vi "ME_acquire_17_DeltaForce_Daq_SteppingMode.vi"() -> ()   [LabVIEW 2015]
doc: "Use this template to build a producer/consumer design pattern. Use this template when you need to execute a process, such as data analysis, when a data source, such as a triggered acquisition, produces data at an uneven rate and you need to execute the process when the data becomes available."
uses:
  Mode.ctl
  oxford_driver/Oxford Drivers/BUSGEN.LLB/OxfordAddress.ctl
  <vilib>/Analysis/baseanly.llb/Mean (DBL).vi
  <vilib>/DAQmx/read.llb/DAQmx Read (Analog 1D DBL 1Chan NSamp).vi
  <vilib>/DAQmx/create/channels.llb/DAQmx Create Channel (AI-Voltage-Basic).vi
  <vilib>/DAQmx/configure/timing.llb/DAQmx Timing (Sample Clock).vi
  <vilib>/Utility/file.llb/Write Delimited Spreadsheet (DBL).vi
  <vilib>/DAQmx/miscellaneous.llb/DAQmx Fill In Error Info.vi
  <vilib>/express/express arith-compare/Formula/XNode/ExpressFormulaBlockNode.xnode
  <vilib>/Analysis/NI_AALBase.lvlib
panel:
  in  "First Offset?":bool
  out "Last2":dbl
  out "Actual2":dbl
  out "Up/Down":bool
  out "T array":dbl[](array[numeric])
  out "Averaged I(T)":dbl[][](array[numeric])
  in  "Averaged P(T)":dbl[][](array[numeric])
  out "remaining elements 2":T1(array[cluster])
  out "Actual mean":dbl format="%0.6f"
  in  "Averaged dt":dbl[][](array[numeric])
  in  "Averaged P(B)":dbl[][](array[numeric])
  out "LockInR":dbl
  out "deltaUaux":dbl
  out "Actual Voltage (V)":dbl caption="Actual AuxV" step=0.1
  in  "Stop":bool
  out "SaveSweep":bool=TRUE
  out "Measurement File_dn":path
  out "Measurement File_up":path
  out "Measurement File_average":path
  out "Actual Polarization":dbl
  in  "Reset IB?":bool
  in  "First?":bool
  in  "Save Period":dbl=1.0
  out "Averaged I(B)":dbl[][](array[numeric])
  out "P(uC/mm^2)":dbl[](array[numeric])
  in  "Sweep":bool
  out "Offset array":dbl[](array[numeric])
  in  "stop 2":bool
  in  "dB":dbl=0.005
  out "appended array":dbl[][](array[numeric])
  out "Actual B Field (T)":dbl
  out "Actual Temperature (K)":dbl
  out "Actual Current (pA)":dbl
  in  "Tab Control":T2(tab)
  in  "dt (K)":dbl=0.1
  in  "Max temperature (K)":dbl=20.0
  in  "Min Temperature (K)":dbl=4.5
  out "P(T)":cluster{dbl[], dbl[]}[](graph)
  out "I(T)":cluster{dbl[], dbl[]}[](graph)
  in  "Set temperature (K)":dbl=4.5
  in  "Temp Ramping Rate (K/min)":dbl=10.0
  in  "Heater Range":enum16{"Off", "Low", "Medium", "High"}(ring)
  in  "Heater On/Off":bool
  out "Setpoint Temperature (K)":dbl
  out "I(T) /Averaged/":cluster{"B array":dbl[], dbl[]}[](graph)
  out "P(T) /Averaged/":cluster{"B array":dbl[], dbl[]}[](graph)
  out "I(B) 3":cluster{dbl[], dbl[]}[](graph)
  out "I(B) /Averaged/":cluster{"B array":dbl[], dbl[]}[](graph)
  out "P(B) /Averaged/":cluster{"B array":dbl[], dbl[]}[](graph)
  out "P(B)":cluster{"yi":dbl[], dbl[]}(graph)
  in  "Set Field (T)":dbl
  in  "Go to Set":bool
  in  "Sweep Rate (T/min)":dbl=2.0 format="%.6f"
  in  "Field To Zero":bool
  out "Target Field":dbl
  in  "Min Field (T)":dbl
  in  "Max Field (T)":dbl=0.15
  in  "Threshold B (T)":dbl
  in  "ReOffset":bool
  in  "Window (s)":dbl
  in  "Field Step (T)":dbl
  in  "Stepping Mode":bool
  out "Ready2Step":bool
  in  "Dwell Time (s)":dbl
  out "B(t)":dbl(graph)
  out "I(t)":dbl(graph)
  out "P(t)":dbl(graph)
  in  "Max count array":i32[](array[numeric])=[2]
  in  "Magnetic Field array (T)":dbl[](array[numeric])=[0.025, 0.05, 0.075, 0.1, 0.125, 0.15, 0.175, 0.2, 0.225, 0.25, 0.275, 0.3]
  in  "T Sweep Rate Array":dbl[](array[numeric])=[10.0, 20.0]
  in  "secs to wait":dbl=180.0
  out "Wait (s)":dbl
  in  "Directory":string
  out "Finished":bool=TRUE
  out "Step Rate":bool
  out "New":bool=TRUE
  in  "Temperature Array":dbl[](array[numeric])=[4.5, 5.0, 6.0, 7.0, 8.0, 9.0, 10.0, 11.0, 12.0]
  in  "Sweep Rate Array":dbl[](array[numeric])=[2.0, 1.0, 0.5, 0.1, 0.05, 9.0, 10.0, 11.0, 12.0]
  in  "Record ALL":bool
  in  "Max Countl":i32
  out "i":i32
  out "j":i32
  out "Step Temp":bool
  in  "FileName":string
  in  "Measure Noise":bool
  in  "Cycles":i32
  in  "maximum value":dbl=10.0 format="%0.2f"
  in  "minimum value":dbl=-10.0 format="%0.2f"
  in  "physical channels":tag="Dev1/ai1"
  out "PSD (pA/Hz^1/2) Peaks Removed":cluster{"f0":dbl, "df":dbl, "magnitude":dbl[]}(graph)
  out "PSD (pA/Hz^1/2)":cluster{"f0":dbl, "df":dbl, "magnitude":dbl[]}(graph)
  out "Current (pA) Filtered":waveform(dbl)(graph)
  out "Current (pA)":dbl[](graph)
  in  "Samples per channel":i32=1000
  in  "Rate":dbl=1000.0 format="%0.2f"
  in  "Cut-Off Frequency":dbl=100.0 caption="Lower Cut-Off"
  in  "Filter On":bool
  in  "Count":i32=60
  in  "Keithley (IV conv) averaging":i32=10
  in  "Lock_in_Amplifier":refnum<visa-resource-name>="GPIB0::5::INSTR"
  out "Dc offset":dbl
  in  "Calibrate":bool
  in  "IV converter":refnum<visa-resource-name>="GPIB0::20::INSTR"
  in  "Magnetic Field":refnum<visa-resource-name>="GPIB0::21::INSTR"
  out "Time Lag":dbl=0.0500025749206543
  in  "Lake Shore":refnum<visa-resource-name>="GPIB0::11::INSTR"
  in  "Temp Refresh (s)":dbl=0.1
  in  "Sampling rate (Hz)":dbl=10.0
  in  "Gain (V/A)":dbl=1000000000.0
  in  "Sample area (mm^2)":dbl=1.0
  out "B_V":cluster{dbl[], "Best Linear Fit":dbl[]}[](graph)=[{[-0.00769241141, -0.00768011662, -0.0029394633, 0.00271952438, 0.00937200583, 0.0154641889, 0.0217080684, 0.0281692221, 0.0344763397, 0.0407091529, 0.0473661569, 0.0541476438, 0.0611164384, 0.0676637725, 0.073937413, 0.0801511723, 0.0863882257, 0.0933787866, 0.0997676928, 0.106163316, 0.113953626, 0.118979018, 0.126030157, 0.132855724, 0.13883398, 0.14631074, 0.153030676, 0.159156864, 0.165801088, 0.17248087, 0.178555009, 0.185285367, 0.192834407, 0.198751051, 0.205413053, 0.212847389, 0.219477697, 0.225574642, 0.232225854, 0.239015189, 0.245675966, 0.252411162, 0.258453848, 0.265211852, 0.271251534, 0.277801221, 0.284008329, 0.291402813, 0.297970768, 0.304082546, 0.310761405, 0.317366634, 0.323522001, 0.330123184, 0.336841279, 0.343557963, 0.349608435, 0.356238003, 0.363590921, 0.370338319, 0.376962983], "Best Linear Fit"=[0.0, 0.0015, 0.0035, 0.0056, 0.0076, 0.0096, 0.0116, 0.0136, 0.0156, 0.0177, 0.0197, 0.0219, 0.0239, 0.0259, 0.0279, 0.0299, 0.032, 0.034, 0.036, 0.038, 0.04, 0.042, 0.0441, 0.046, 0.048, 0.05, 0.052, 0.054, 0.056, 0.058, 0.06, 0.0621, 0.0643, 0.0663, 0.0684, 0.0704, 0.0725, 0.0745, 0.0765, 0.0787, 0.0807, 0.0827, 0.0847, 0.0868, 0.0888, 0.0908, 0.0928, 0.0948, 0.0968, 0.0988, 0.1008, 0.1028, 0.1048, 0.1069, 0.1091, 0.1111, 0.1131, 0.1152, 0.1173, 0.1193, 0.1213]}, {[-0.00769241141, -0.00768011662, -0.0029394633, 0.00271952438, 0.00937200583, 0.0154641889, 0.0217080684, 0.0281692221, 0.0344763397, 0.0407091529, 0.0473661569, 0.0541476438, 0.0611164384, 0.0676637725, 0.073937413, 0.0801511723, 0.0863882257, 0.0933787866, 0.0997676928, 0.106163316, 0.113953626, 0.118979018, 0.126030157, 0.132855724, 0.13883398, 0.14631074, 0.153030676, 0.159156864, 0.165801088, 0.17248087, 0.178555009, 0.185285367, 0.192834407, 0.198751051, 0.205413053, 0.212847389, 0.219477697, 0.225574642, 0.232225854, 0.239015189, 0.245675966, 0.252411162, 0.258453848, 0.265211852, 0.271251534, 0.277801221, 0.284008329, 0.291402813, 0.297970768, 0.304082546, 0.310761405, 0.317366634, 0.323522001, 0.330123184, 0.336841279, 0.343557963, 0.349608435, 0.356238003, 0.363590921, 0.370338319, 0.376962983], "Best Linear Fit"=[0.002353460844818253, 0.002357267374965663, 0.003824997997530172, 0.005577049655813272, 0.007636692089275871, 0.009522863265806463, 0.01145600043639222, 0.013456406815525209, 0.015409122826751182, 0.01733883381400479, 0.019399876452181594, 0.021499459635718428, 0.023657034245452215, 0.025684122519169482, 0.027626473848249778, 0.02955028565017564, 0.03148130942513291, 0.03364562299316916, 0.03562366117513693, 0.037603778974812686, 0.040015698972850115, 0.04157158615356273, 0.04375465501257369, 0.04586788562152819, 0.0477187843918964, 0.050033627699098075, 0.05211415440778254, 0.05401085368533849, 0.056067939569859164, 0.05813603439385595, 0.06001661903361471, 0.06210037244704129, 0.06443759401357516, 0.0662694173922171, 0.06833200743687069, 0.07063371605572277, 0.07268649347515121, 0.0745741389696738, 0.07663338837489471, 0.07873540137051047, 0.08079761214887074, 0.08288286343195213, 0.08475371006132383, 0.08684602281837933, 0.08871593939391825, 0.09074375613756333, 0.09266550866283872, 0.09495487889775463, 0.09698835150804998, 0.09888058937557581, 0.10094839843403076, 0.10299341126621803, 0.10489914451207855, 0.10694290468187984, 0.10902286140750632, 0.11110238128028392, 0.11297563849525552, 0.11502818680688229, 0.1173046879946565, 0.11939371707962458, 0.12144474708765744]}]
  out "V_I":cluster{dbl[], "Best Linear Fit":dbl[]}[](graph)=[{[0.0, 0.012, 0.026, 0.04, 0.054, 0.068, 0.081, 0.096, 0.11, 0.124, 0.138, 0.153, 0.167, 0.18, 0.195, 0.208, 0.223, 0.236, 0.251, 0.265, 0.279, 0.292, 0.306, 0.32, 0.334, 0.348, 0.362, 0.375, 0.389, 0.403, 0.417, 0.432, 0.446, 0.46, 0.475, 0.489, 0.504, 0.517, 0.531, 0.546, 0.56, 0.574, 0.588, 0.602, 0.616, 0.63, 0.644, 0.658, 0.672, 0.685, 0.699, 0.713, 0.727, 0.742, 0.755, 0.77, 0.784, 0.799, 0.814, 0.827, 0.841], "Best Linear Fit"=[-0.00769241141, -0.00768011662, -0.0029394633, 0.00271952438, 0.00937200583, 0.0154641889, 0.0217080684, 0.0281692221, 0.0344763397, 0.0407091529, 0.0473661569, 0.0541476438, 0.0611164384, 0.0676637725, 0.073937413, 0.0801511723, 0.0863882257, 0.0933787866, 0.0997676928, 0.106163316, 0.113953626, 0.118979018, 0.126030157, 0.132855724, 0.13883398, 0.14631074, 0.153030676, 0.159156864, 0.165801088, 0.17248087, 0.178555009, 0.185285367, 0.192834407, 0.198751051, 0.205413053, 0.212847389, 0.219477697, 0.225574642, 0.232225854, 0.239015189, 0.245675966, 0.252411162, 0.258453848, 0.265211852, 0.271251534, 0.277801221, 0.284008329, 0.291402813, 0.297970768, 0.304082546, 0.310761405, 0.317366634, 0.323522001, 0.330123184, 0.336841279, 0.343557963, 0.349608435, 0.356238003, 0.363590921, 0.370338319, 0.376962983]}, {[0.0, 0.012, 0.026, 0.04, 0.054, 0.068, 0.081, 0.096, 0.11, 0.124, 0.138, 0.153, 0.167, 0.18, 0.195, 0.208, 0.223, 0.236, 0.251, 0.265, 0.279, 0.292, 0.306, 0.32, 0.334, 0.348, 0.362, 0.375, 0.389, 0.403, 0.417, 0.432, 0.446, 0.46, 0.475, 0.489, 0.504, 0.517, 0.531, 0.546, 0.56, 0.574, 0.588, 0.602, 0.616, 0.63, 0.644, 0.658, 0.672, 0.685, 0.699, 0.713, 0.727, 0.742, 0.755, 0.77, 0.784, 0.799, 0.814, 0.827, 0.841], "Best Linear Fit"=[-0.015941127780698654, -0.010342478990544012, -0.0038107220686969304, 0.0027210348531501527, 0.009252791774997235, 0.01578454869684432, 0.02184975155284518, 0.028848062540538483, 0.03537981946238557, 0.041911576384232645, 0.048443333306079736, 0.05544164429377303, 0.061973401215620116, 0.06803860407162098, 0.07503691505931429, 0.08110211791531513, 0.08810042890300844, 0.0941656317590093, 0.10116394274670261, 0.1076956996685497, 0.11422745659039678, 0.12029265944639762, 0.1268244163682447, 0.1333561732900918, 0.13988793021193888, 0.14641968713378595, 0.15295144405563305, 0.15901664691163392, 0.165548403833481, 0.1720801607553281, 0.17861191767717516, 0.18561022866486845, 0.19214198558671555, 0.19867374250856262, 0.20567205349625592, 0.212203810418103, 0.2192021214057963, 0.22526732426179719, 0.23179908118364426, 0.23879739217133758, 0.24532914909318465, 0.2518609060150317, 0.2583926629368788, 0.2649244198587259, 0.271456176780573, 0.27798793370242003, 0.28451969062426713, 0.29105144754611423, 0.2975832044679613, 0.3036484073239622, 0.31018016424580924, 0.3167119211676563, 0.3232436780895034, 0.3302419890771967, 0.3363071919331976, 0.3433055029208909, 0.34983725984273795, 0.35683557083043127, 0.36383388181812454, 0.3698990846741254, 0.3764308415959725]}]
  out "B0 (T)":dbl=0.0026443907573365636
  out "B/V (T/V)":dbl=0.3027997253900218
  out "I0 (A)":dbl=-0.008736391445912099
  out "V/I (Ohm)":dbl=0.4773805959957447
  in  "Offset?":bool
  in  "Magnet":bool=TRUE
  in  "Ramp":bool=TRUE
  in  "DaQ":bool
  in  "Moving average":i8=10
  in  "Sample Rate":dbl=1000.0
  in  "Number of Samples":i32=100
  in  "Physical Channel":tag="kartya/ai0"
  in  "Min Voltage":dbl=-5.0
  in  "Max Voltage":dbl=5.0
  in  "Terminal Configuration":i32(ring)=-1 items=["default"=-1, "RSE"=10083, "NRSE"=10078, "Differential"=10106, "Pseudodifferential"=12529]
  out "Confirm":bool
  in  "Dwell Time (ms)":u32=1000
  in  "Temp/Magnetic Field":bool
  out "index":i8
  out "Read?":bool
  out "Magnetic Field (T)":dbl[](array[numeric])
  out "Reset":bool
  out "Measured Current (pA)":dbl[](array[numeric])
  out "Elapsed Time (s)":dbl[](array[numeric])
  out "Start time":timestamp
  in  "Enum":T3=enum."Process"
  out "B array":dbl[](array[numeric])
  in  "dB (T)":dbl=0.0025
  in  "Counter":i8
  out "L magnet (H)":dbl
  out "R magnet (mOhm)":dbl
  out "Actual Current (R0)":dbl
  out "Actual Field (T)":dbl
  out "Temperature array":dbl[](array[numeric])
  in  "New Measurement File":bool
  out "Measurement File":path
  out "refnum out":refnum<file>
  in  "Measuring":bool
  in  "Measure /Pause":bool
  in  "stop":bool
  # "DeltaForce"
  # "Discrete"
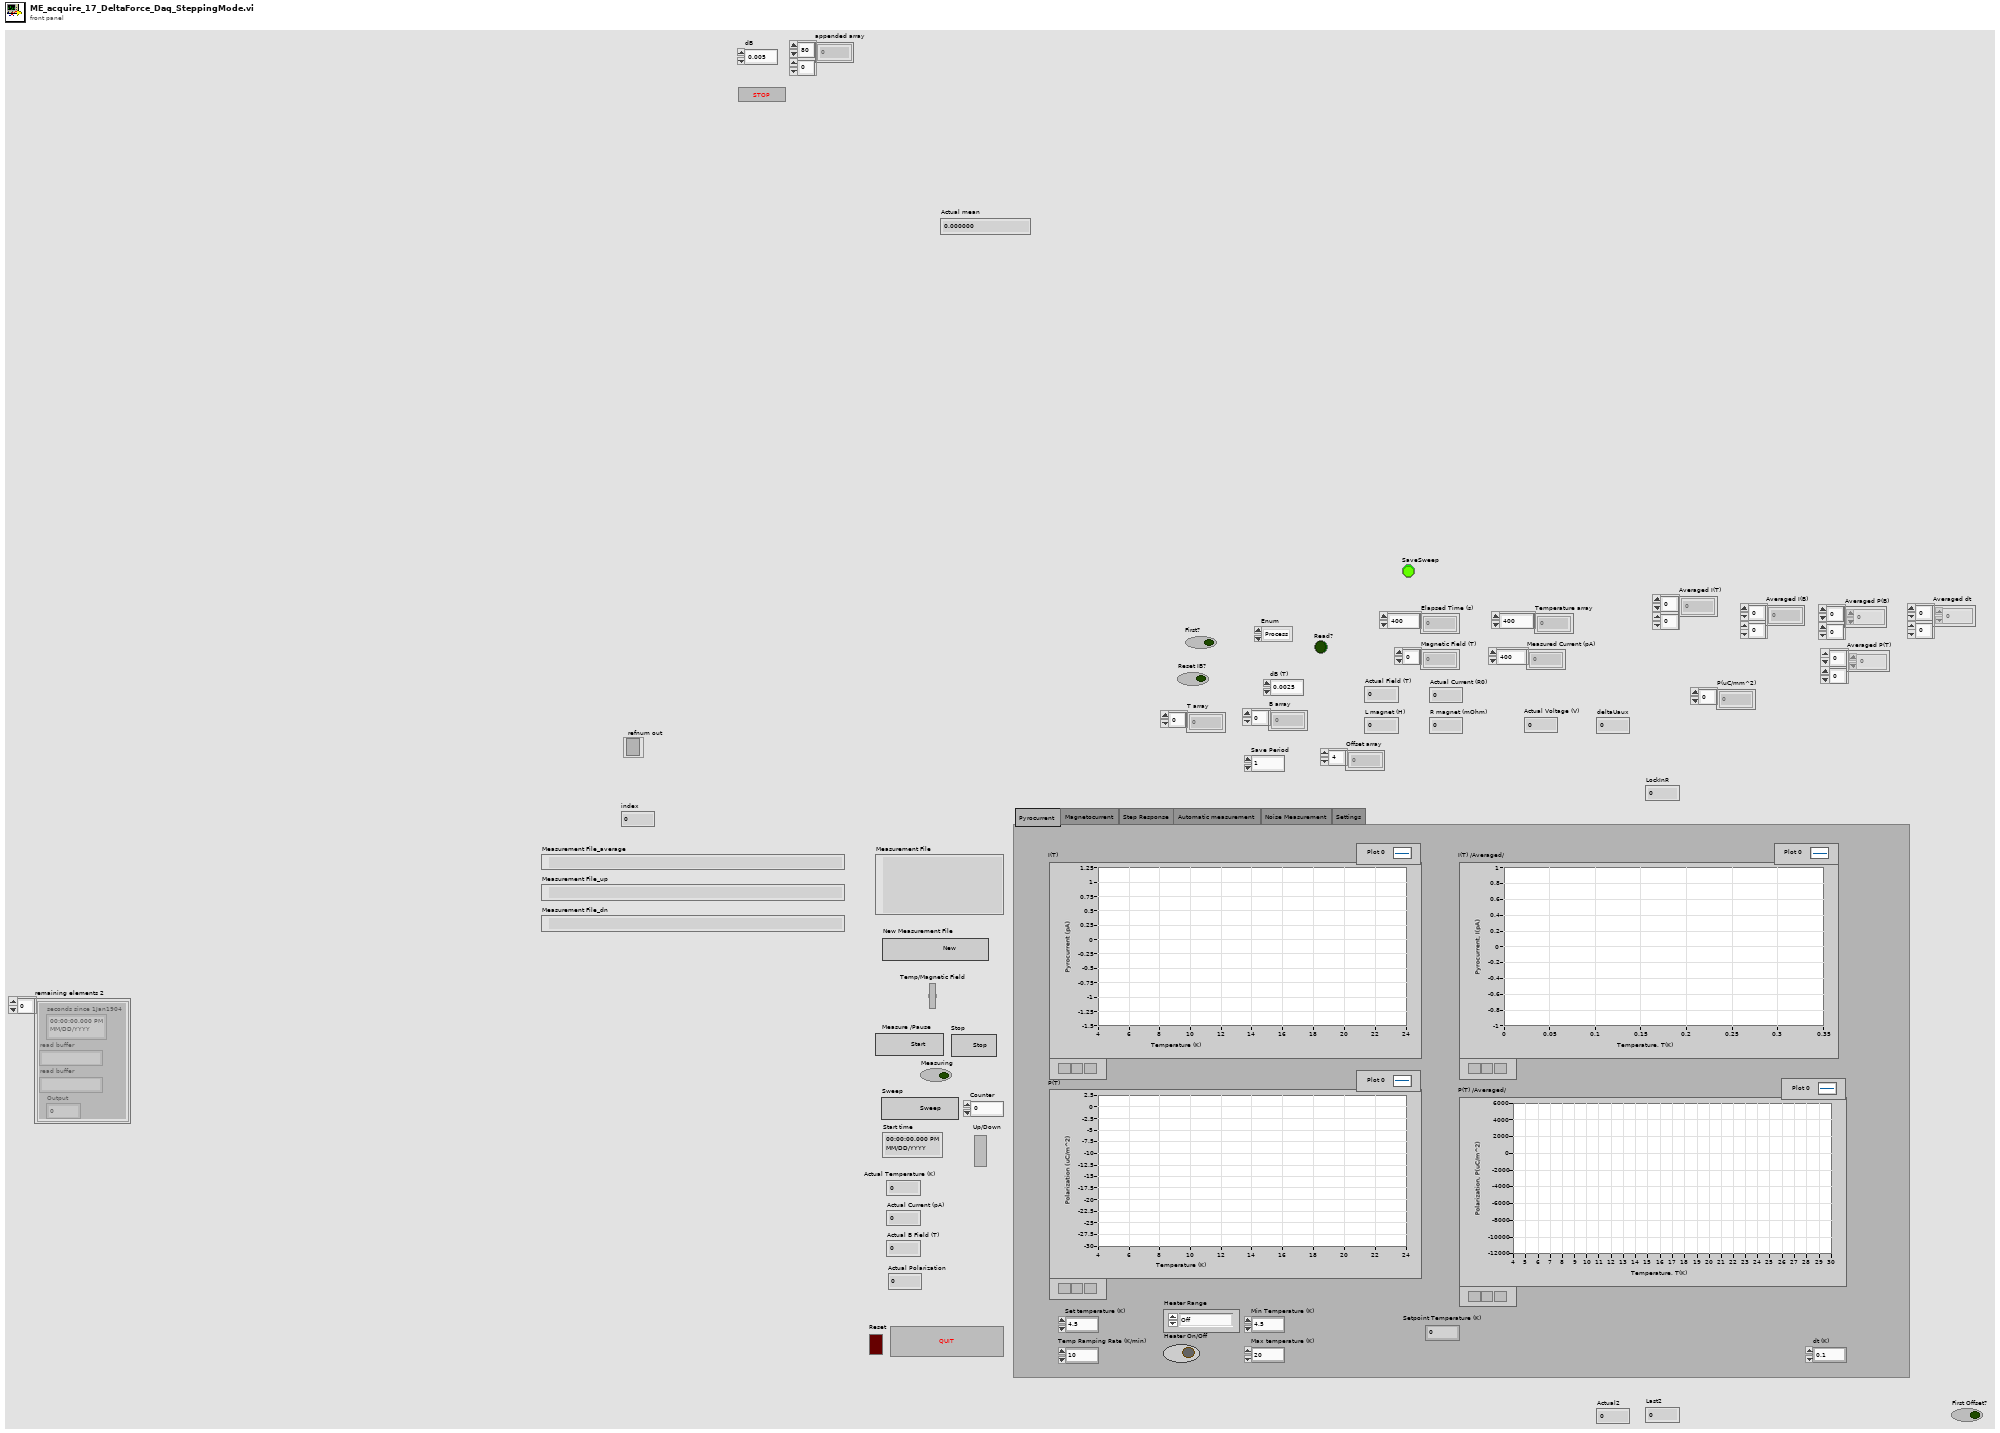
[diagram p1: front panel]
types:
  T1 = cluster{"seconds since 1Jan1904":timestamp, "read buffer":string, "read buffer":string, "Output":dbl}[]
  T2 = enum32{"Pyrocurrent", "Magnetocurrent", "Step Response", "Automatic measurement", "Noise Measurement", "Settings"}
  T3 = typedef "Mode.ctl" = enum16{"Offset", "Process", "Sweep", "StepOxford", "StepDelta", "Plot", "Save", "New", "Return", ""}
  T4 = cluster{"seconds since 1Jan1904":timestamp, "read buffer":string, "read buffer":string, "Output":dbl}
  T5 = enum16{"open", "replace", "create", "open or create", "replace or create", "replace or create with confirmation"}
  T6 = typedef "OxfordAddress.ctl" = cluster{"Com Port":i32, "ISOBUS Address":i32, "GPIB Address":i16, "Communication":enum16{"RS232", "ISOBUS", "GPIB", "Gateway"}}
  T7 = cluster{"B array":dbl[], "Averaged P(B) Out":dbl[]}
  T8 = cluster{"B array":dbl[], "BaselineSubtracted I(B)":dbl[]}
  T9 = cluster{"B array":dbl[], "Averaged P(B) Out":dbl[]}[]
  T10 = cluster{"B array":dbl[], "BaselineSubtracted I(B)":dbl[]}[]
  T11 = cluster{"T array":dbl[], "Averaged P(T) Out":dbl[]}
  T12 = cluster{"T array":dbl[], "Averaged I(B) out":dbl[]}
  T13 = cluster{"T array":dbl[], "Averaged P(T) Out":dbl[]}[]
  T14 = cluster{"T array":dbl[], "Averaged I(B) out":dbl[]}[]
  T15 = cluster{"I array out (A)":dbl[], "V array out (V)":dbl[]}
  T16 = cluster{"I array out (A)":dbl[], "Best Linear Fit":dbl[]}
  T17 = cluster{"V array out (V)":dbl[], "B array Out":dbl[]}
  T18 = cluster{"V array out (V)":dbl[], "Best Linear Fit 2":dbl[]}
  T19 = cluster{"I array out (A)":dbl[], "Best Linear Fit":dbl[]}[]
  T20 = cluster{"V array out (V)":dbl[], "Best Linear Fit 2":dbl[]}[]
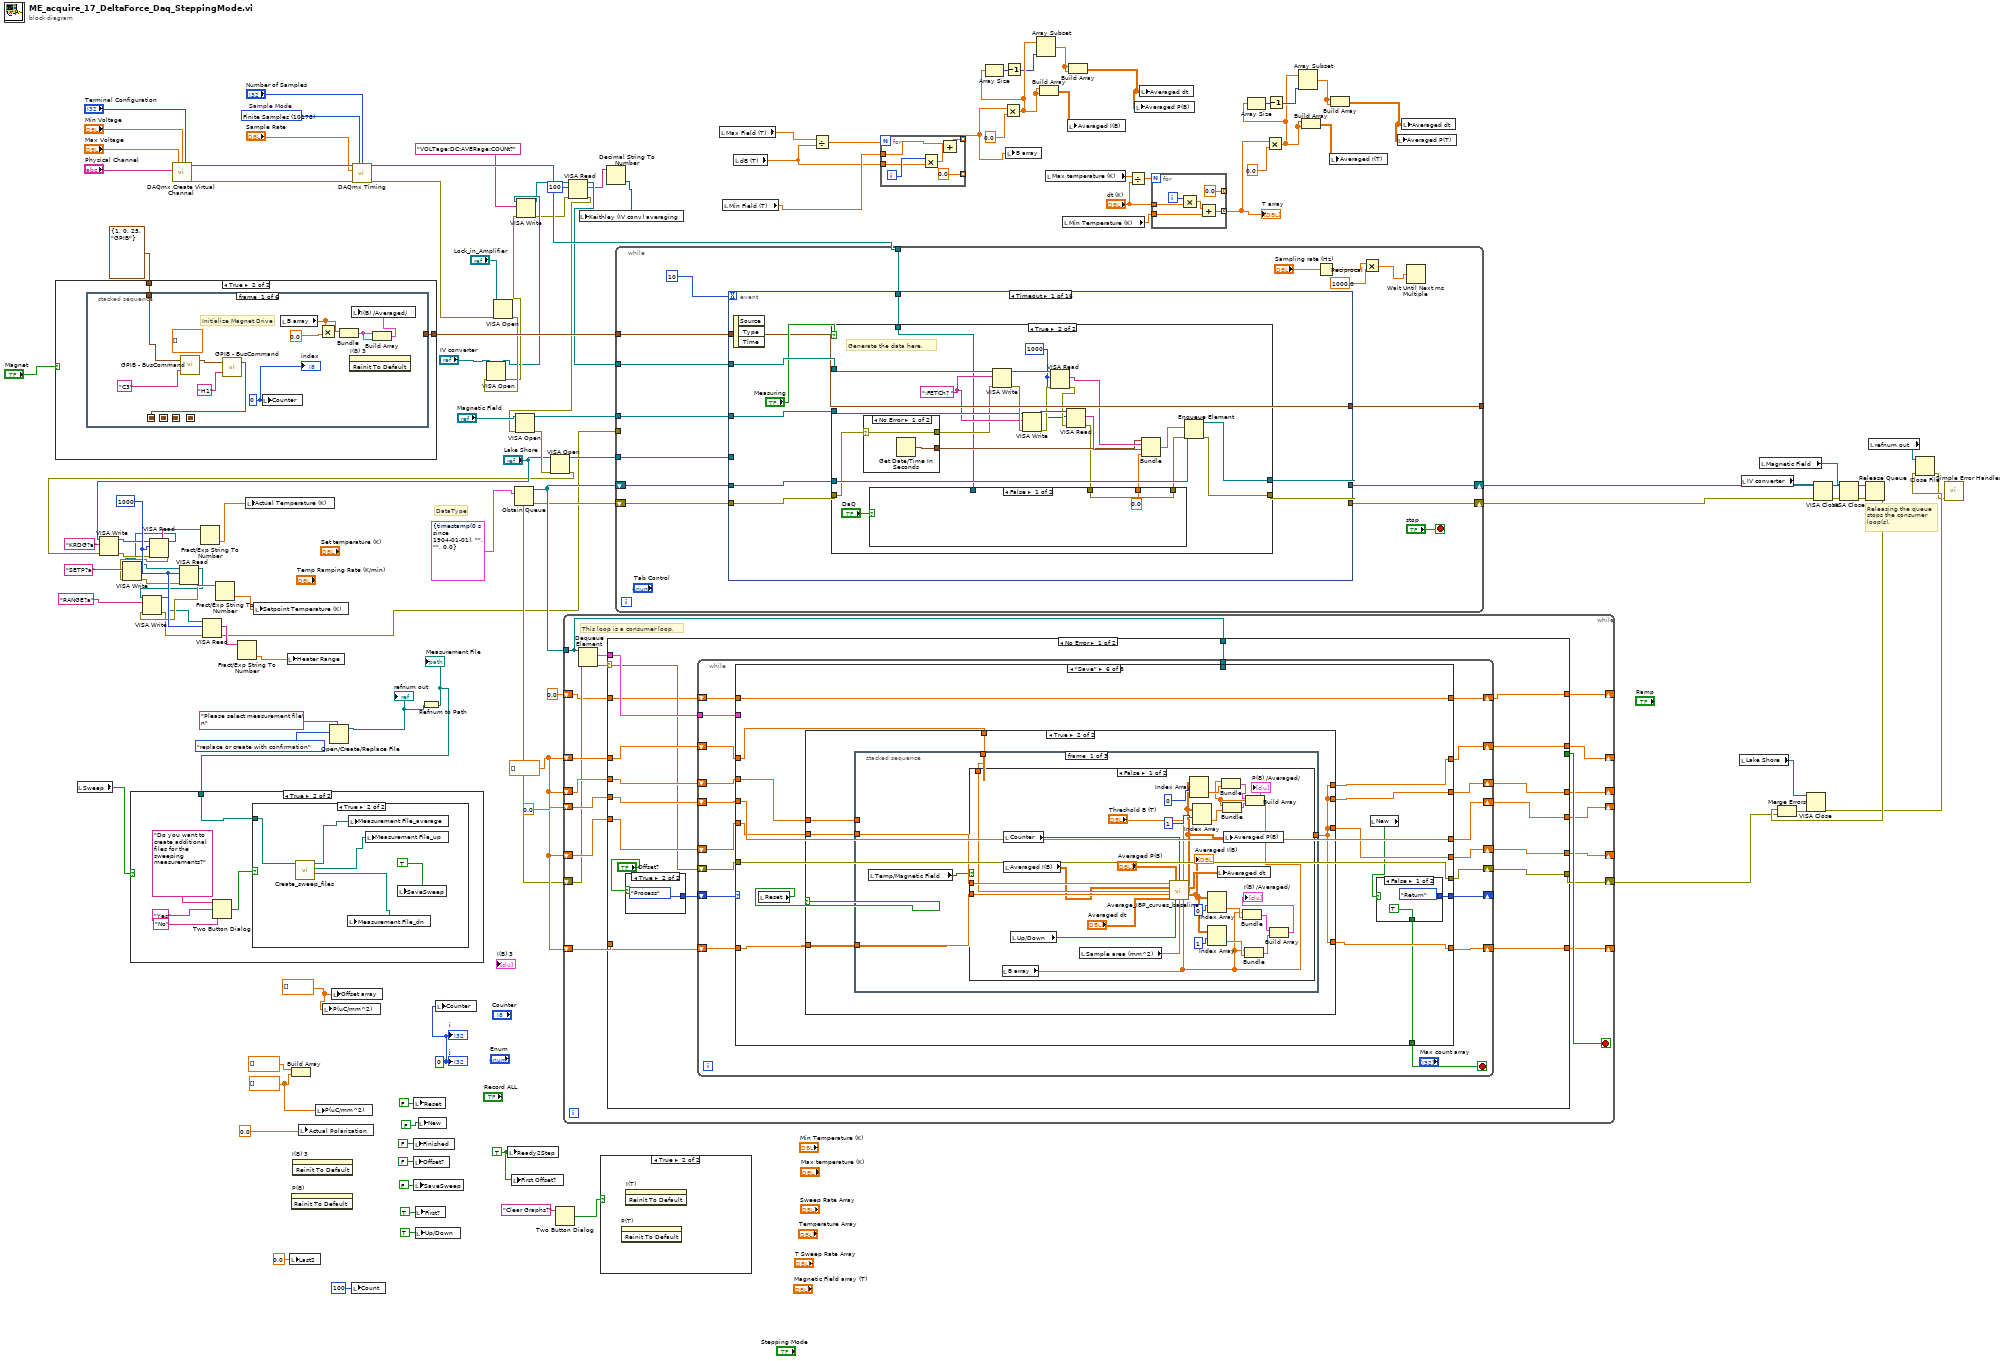
[diagram p0: block diagram]
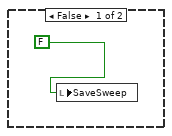
[diagram p4: hidden frame]
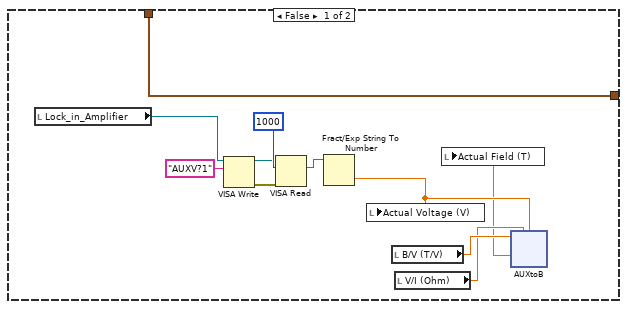
[diagram p5: hidden frame]
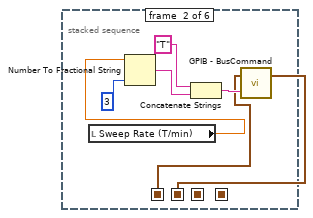
[diagram p6: hidden frame]
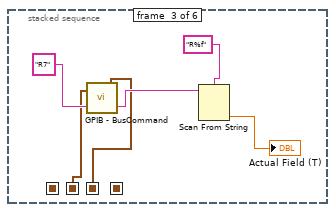
[diagram p7: hidden frame]
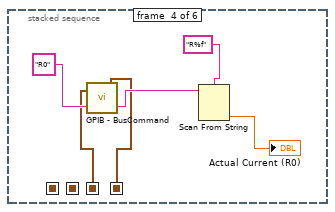
[diagram p8: hidden frame]
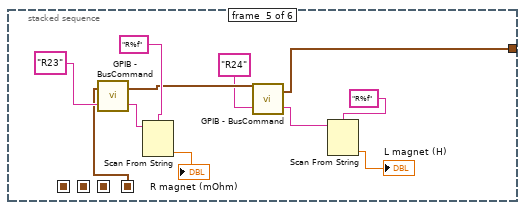
[diagram p9: hidden frame]
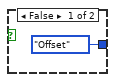
[diagram p11: hidden frame]
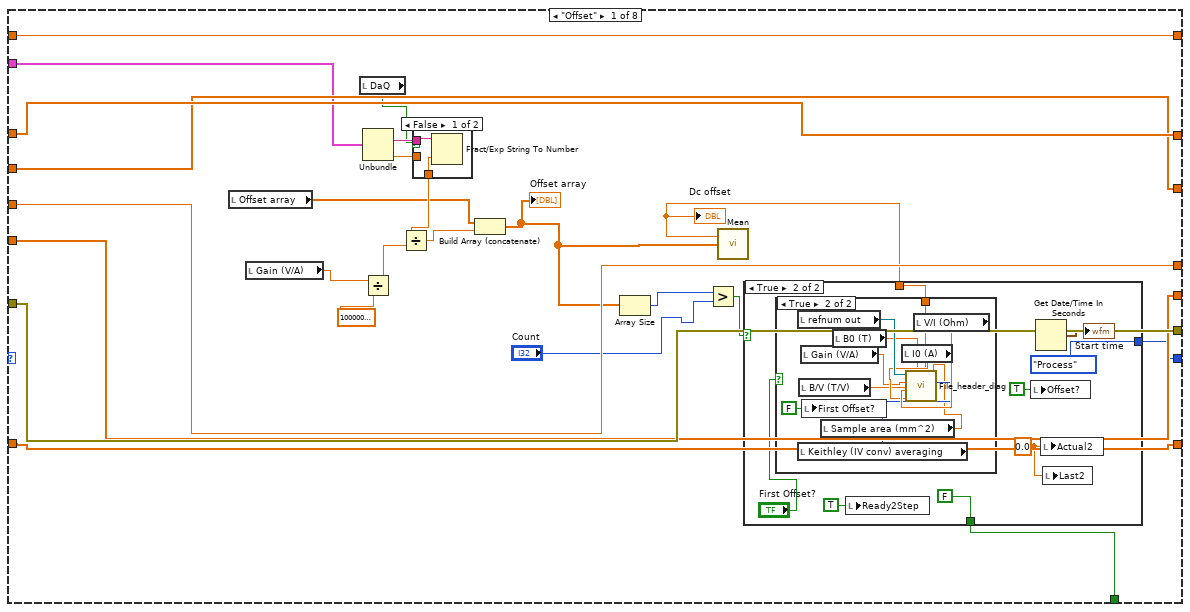
[diagram p12: hidden frame]
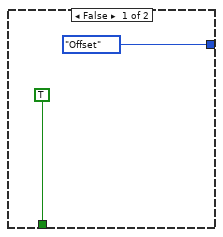
[diagram p14: hidden frame]
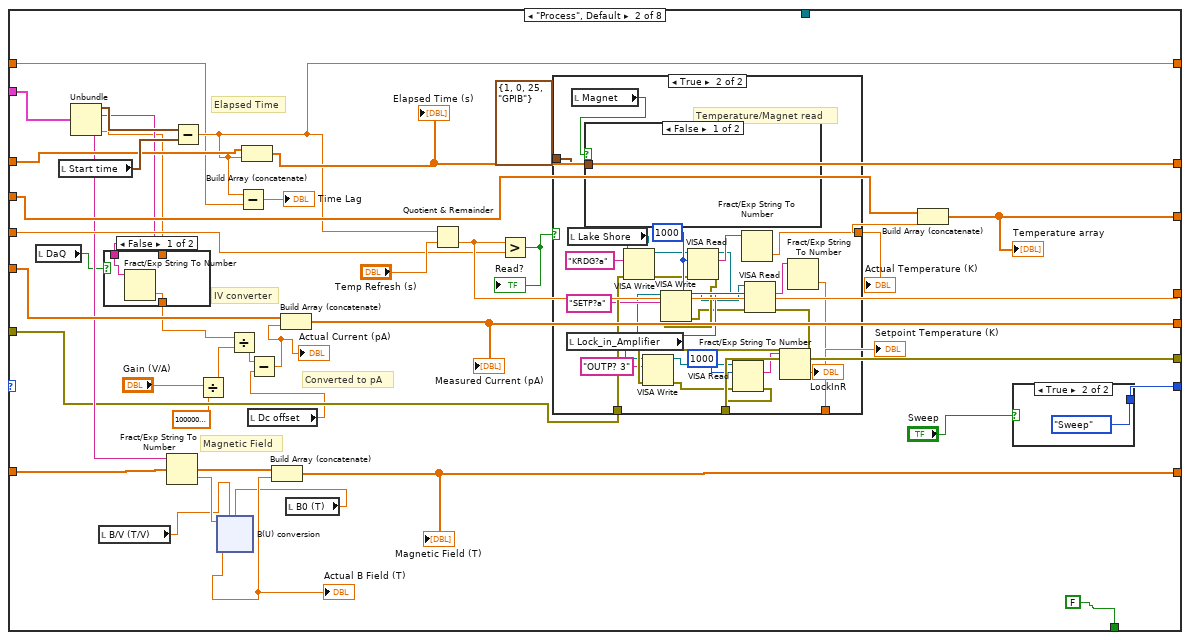
[diagram p16: hidden frame]
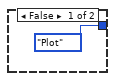
[diagram p18: hidden frame]
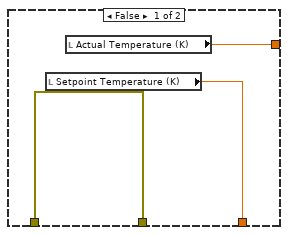
[diagram p19: hidden frame]
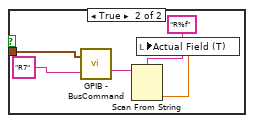
[diagram p20: hidden frame]
diagram:
  w3 = TRUE ("Ready2Step")
  w38 = 10178 items=["Finite Samples"=10178, "Continuous Samples"=10123, "Hardware Timed Single Point"=12522]  # Sample Mode
  w65 = u32 1000 ("byte count")
  w76 = 0 ("j")
  w73 = dbl[] []
  w90 = dbl[] []
  w96 = dbl[] []
  # "DataType"
  # "Releasing the queue stops the consumer loop(s)."
  n1 = case shown="True" "Magnet" {
    tunnel: T6 {"Com Port"=1, "ISOBUS Address"=0, "GPIB Address"=25, "Communication"=enum."GPIB"} ("Address") -> [w130 w144]
    tunnel: [w130 w143] -> w102
    frame False {
      n2 = local read "Lock_in_Amplifier"() -> (w124:refnum<visa-resource-name>)
      n3 = VISA Write(VISA resource name=w124, write buffer="AUXV?1") -> (VISA resource name out=w125:refnum<visa-resource-name>, error out=w129:errorcluster)  [unwired: 1 in, 1 out]
      n4 = VISA Read(VISA resource name=w125, byte count=u32 1000, error in (no error)=w129) -> (read buffer=w128:string)  [unwired: 3 out]
      n5 = Fract/Exp String To Number(string=w128) -> (number=w121:dbl)  [unwired: 3 in, 1 out]
      n6 = local write "Actual Voltage (V)"(w121) -> ()
      n7 = local read "B/V (T/V)"() -> (w123:dbl)
      n8 = local read "V/I (Ohm)"() -> (w122:dbl)
      n9 = xnode "AUXtoB"("BpV"=w123, "Rm"=w122, "Aux"=w121) -> ("Result"=w120:dbl)  [unwired: 1 in, 1 out]
      n10 = local write "Actual Field (T)"(w120) -> ()
    }
    frame True {
      n11 = stacked-sequence {
        seq-local: [w152 _ _ _ _ _] -> [_ w157 _ _ _ _]
        seq-local: [_ w156 _ _ _ _] -> [_ _ w164 _ _ _]
        seq-local: [_ _ w163 _ _ _] -> [_ _ _ w170 _ _]
        seq-local: [_ _ _ w169 _ _] -> [_ _ _ _ w181 _]
        tunnel: w144 -> [w154 _ _ _ _ _]
        tunnel: [_ _ _ _ w179 _] -> w143
        frame #0 {
          (unwired) dbl[][] []
          w150 = i8 0 ("Counter")
          # "Initialize Magnet Drive"
          n12 = call "GPIB - BusCommand.vi"("Command"="C3", "Address"=w154) -> ("Address(thru)"=w153:T6)  [unwired: 1 out]
          n13 = call "GPIB - BusCommand.vi"("Command"="H1", "Address"=w153) -> ("Address(thru)"=w152:T6)  [unwired: 1 out]
          n14 = local write "Counter"(w150) -> ()
          n15 = local read "B array"() -> (w148:dbl[])
          n16 = Multiply(x=w148, y=0.0) -> (x*y=w147:dbl[])
          n17 = Bundle("B array"=w148, w147) -> (w146:cluster{"B array":dbl[], dbl[]})  [unwired: 1 in]
          n18 = invoke on="I(B) 3" class="XYGraph (strict)" method="Reinit To Default"() -> ()  [unwired: 3 in, 3 out]
          n19 = Build Array(w146, w146) -> (w145:cluster{"B array":dbl[], dbl[]}[])
          n20 = local write "I(B) /Averaged/"(w145) -> ()
          "index" <- w150
        }
        frame #1 {
          n21 = local read "Sweep Rate (T/min)"() -> (w158:dbl)
          n22 = Number To Fractional String(number=w158, precision (6)=i16 3) -> (F-format string=w160:string)  [unwired: 2 in]
          n23 = Concatenate Strings("T" ("format string"), w160) -> (w159:string)
          n24 = call "GPIB - BusCommand.vi"("Command"=w159, "Address"=w157) -> ("Address(thru)"=w156:T6)  [unwired: 1 out]
        }
        frame #2 {
          n25 = call "GPIB - BusCommand.vi"("Command"="R7" ("format string"), "Address"=w164) -> ("Reply"=w168:string, "Address(thru)"=w163:T6)
          n26 = Scan From String(format string="R%f" ("remaining string"), input string=w168) -> (output 1=→"Actual Field (T)":dbl)  [unwired: 3 in, 3 out]
        }
        frame #3 {
          n27 = call "GPIB - BusCommand.vi"("Command"="R0" ("format string"), "Address"=w170) -> ("Reply"=w174:string, "Address(thru)"=w169:T6)
          n28 = Scan From String(format string="R%f" ("remaining string"), input string=w174) -> (output 1=→"Actual Current (R0)":dbl)  [unwired: 3 in, 3 out]
        }
        frame #4 {
          n29 = call "GPIB - BusCommand.vi"("Command"="R23" ("format string"), "Address"=w181) -> ("Reply"=w185:string, "Address(thru)"=w180:T6)
          n30 = Scan From String(format string="R%f" ("remaining string"), input string=w185) -> (output 1=→"R magnet (mOhm)":dbl)  [unwired: 3 in, 3 out]
          n31 = call "GPIB - BusCommand.vi"("Command"="R24" ("format string"), "Address"=w180) -> ("Reply"=w177:string, "Address(thru)"=w179:T6)
          n32 = Scan From String(format string="R%f" ("remaining string"), input string=w177) -> (output 1=→"L magnet (H)":dbl)  [unwired: 3 in, 3 out]
        }
        frame #5 {
        }
      }
    }
  }
  n33 = local read "Sweep"() -> (w81:bool)
  n34 = call-poly <vilib>:"DAQmx Create Virtual Channel.vi"("maximum value"="Max Voltage", "minimum value"="Min Voltage", "input terminal configuration"="Terminal Configuration", "physical channels"="Physical Channel") -> ("task out"=w36:refnum<k21>, "error out"=w37:errorcluster)  [unwired: 10 in]
  n35 = local write "Last2"(0.0 ("Last2")) -> ()
  n36 = Build Array(dbl[] [], w73) -> ()  [unwired: 1 out]
  n37 = invoke on="P(B)" class="XYGraph (strict)" method="Reinit To Default"() -> ()  [unwired: 3 in, 3 out]
  n38 = invoke on="I(B) 3" class="XYGraph (strict)" method="Reinit To Default"() -> ()  [unwired: 3 in, 3 out]
  n39 = local write "Actual Polarization"(0.0 ("Actual Polarization")) -> ()
  n40 = local write "P(uC/mm^2)"(w73) -> ()
  n41 = local write "P(uC/mm^2)"(w90) -> ()
  n42 = Open/Create/Replace File(prompt="Please select measurement file\n", operation (0:open)=T5."replace or create with confirmation") -> (refnum out=w99:refnum<file>)  [unwired: 4 in, 2 out]
  "refnum out" <- w99
  n43 = local write "Offset array"(w90) -> ()
  n44 = local write "Count"(100 ("Count")) -> ()
  n45 = call-poly <vilib>:"DAQmx Timing.vi"("task/channels in"=w36, "sample mode"=w38, "samples per channel"="Number of Samples", "rate"="Sample Rate", "error in"=w37) -> ("task out"=w28:refnum<k21>, "error out"=w29:errorcluster)  [unwired: 9 in]
  n46 = local write "Finished"(FALSE ("Finished")) -> ()
  n47 = local write "Offset?"(FALSE ("Offset?")) -> ()
  n48 = local write "Reset"(FALSE ("Reset")) -> ()
  n49 = local write "SaveSweep"(FALSE ("SaveSweep")) -> ()
  n50 = local write "First?"(TRUE ("First?")) -> ()
  n51 = local write "Up/Down"(TRUE ("Up/Down")) -> ()
  n52 = local write "New"(FALSE ("New")) -> ()
  n53 = Refnum to Path(1:w99) -> (0:w80:path)
  "Measurement File" <- w80
  n54 = case shown="True" w81 {
    tunnel: w80 -> [_ w186]
    frame False {
    }
    frame True {
      n55 = Two Button Dialog(message="Do you want to create additional files for the sweeping measurements?" ("string"), 1:"No" ("F button name (\"Cancel\")"), 2:"Yes" ("T button name (\"OK\")")) -> (T button?=w188:bool)
      n56 = case shown="True" w188 {
        tunnel: w186 -> [_ w196]
        frame False {
          n57 = local write "SaveSweep"(FALSE ("SaveSweep")) -> ()
        }
        frame True {
          n58 = call "Create_sweep_files.vi"("Measurement File"=w196) -> ("Path 3"=w193:path, "Path 2"=w194:path, "Path"=w195:path)  [unwired: 8 in]
          n59 = local write "Measurement File_dn"(w193) -> ()
          n60 = local write "Measurement File_average"(w195) -> ()
          n61 = local write "Measurement File_up"(w194) -> ()
          n62 = local write "SaveSweep"(TRUE) -> ()
        }
      }
    }
  }
  n63 = local write "Counter"(w76) -> ()
  n64 = VISA Open(error in (no error)=w29, VISA resource name="Lock_in_Amplifier") -> (error out=w48:errorcluster)  [unwired: 3 in, 1 out]
  n65 = VISA Open(error in (no error)=w48, VISA resource name="IV converter") -> (VISA resource name=w25:refnum<visa-resource-name>, error out=w26:errorcluster)  [unwired: 3 in]
  n66 = local write "Ready2Step"(w3) -> ()
  n67 = local write "First Offset?"(w3) -> ()
  n68 = Obtain Queue(element data type=T4 {"seconds since 1Jan1904"=timestamp(0 s since 1904-01-01), "read buffer"="", "read buffer"="", "Output"=0.0} ("output cluster")) -> (queue out=w119:refnum<queue>, error out=w94:errorcluster)  [unwired: 4 in, 1 out]
  n69 = VISA Write(VISA resource name=w25, write buffer="VOLTage:DC:AVERage:COUNt?", error in (no error)=w26) -> (VISA resource name out=w21:refnum<visa-resource-name>, error out=w23:errorcluster)  [unwired: 1 out]
  n70 = Two Button Dialog(message="Clear Graphs?") -> (T button?=w75:bool)  [unwired: 2 in]
  n71 = while {
    tunnel: w119 -> [w197]
    shift-right: [w210] -> _
    shift-left: w96 -> [w209]
    shift-right: [w208] -> _
    shift-left: w96 -> [w207]
    shift-right: [w206] -> _
    shift-left: w96 -> [w205]
    shift-right: [w204] -> _
    shift-left: 0.0 -> [w203]
    shift-right: [w202] -> _
    shift-left: w96 -> [w201]
    shift-right: [w211] -> w107
    shift-left: w94 -> [w200]
    shift-right: [w199] -> _
    shift-left: 0.0 -> [w198]
    stop <- w212 stop-if-true
    # "This loop is a consumer loop."
    n72 = Dequeue Element(queue=w197, error in (no error)=w200) -> (element=w213:T4, error out=w214:errorcluster)  [unwired: 1 in, 2 out]
    n73 = case shown="No Error" w214 {
      selector: w214 -> [w220 w1123]
      tunnel: w213 -> [w231 _]
      tunnel: [_ TRUE] -> w212
      tunnel: [w219 w1123] -> w211
      tunnel: [w230 w1122] -> w210
      tunnel: w209 -> [w229 w1122]
      tunnel: [w228 w1119] -> w208
      tunnel: w207 -> [w227 w1119]
      tunnel: [w226 w1118] -> w206
      tunnel: w205 -> [w225 w1118]
      tunnel: [w224 w1120] -> w204
      tunnel: w203 -> [w223 w1120]
      tunnel: [w222 w1121] -> w202
      tunnel: w201 -> [w221 w1121]
      tunnel: [w218 w1117] -> w199
      tunnel: w198 -> [w217 w1117]
      tunnel: w197 -> [w215 _]
      frame No Error {
        n74 = case shown="True" "Offset?" {
          tunnel: [Mode."Offset" ("Enum") Mode."Process" ("Enum")] -> w232
          frame False {
          }
          frame True {
          }
        }
        n75 = while {
          shift-right: [w241] -> _
          shift-left: w232 -> [w253]
          tunnel: w231 -> [w252]
          shift-right: [w251] -> w230
          shift-left: w229 -> [w250]
          shift-right: [w243] -> w222
          shift-left: w221 -> [w242]
          shift-right: [w245] -> w224
          shift-left: w223 -> [w244]
          shift-right: [w249] -> w228
          shift-left: w227 -> [w248]
          shift-right: [w239] -> w219
          shift-left: w220 -> [w240]
          shift-right: [w247] -> w226
          shift-left: w225 -> [w246]
          shift-right: [w237] -> w218
          shift-left: w217 -> [w236]
          tunnel: w215 -> [w235]
          stop <- w238 stop-if-true
          n76 = case shown="\"Save\"" w253 {
            selector: w253 -> [_ _ _ _ _ _ _ w1110]
            tunnel: w252 -> [w271 w339 _ _ _ _ _ _]
            tunnel: [w277 w336 w397 w544 w656 w775 w886 w1115] -> w251
            tunnel: w250 -> [w277 w329 w397 w544 w656 w771 w886 w1115]
            tunnel: [w272 w335 w400 w541 w658 w777 w884 w1112] -> w249
            tunnel: w248 -> [w272 w334 w400 w541 w658 w772 w884 w1112]
            tunnel: [w273 w333 w402 w540 w653 w778 w882 w1109] -> w247
            tunnel: w246 -> [w273 w332 w402 w540 w653 w773 w882 w1109]
            tunnel: [w275 w328 w399 w542 w654 w781 0.0 w1113] -> w245
            tunnel: w244 -> [w275 w327 w399 w542 w654 w781 _ w1113]
            tunnel: [w276 w324 w398 w543 w655 w776 w885 w1114] -> w243
            tunnel: w242 -> [w276 w325 w398 w543 w655 w774 w885 w1114]
            tunnel: [w261 w322 w395 w534 Mode."Save" ("Enum") w782 Mode."Return" ("Enum") w1110] -> w241
            tunnel: w240 -> [w274 w320 w404 w538 w661 w780 w878 w1111]
            tunnel: [w274 w319 w403 w537 w661 w780 w877 w1111] -> w239
            tunnel: [w257 FALSE FALSE FALSE FALSE w769 TRUE TRUE] -> w238
            tunnel: [w260 w316 w396 w535 w657 w779 0.0 w1116] -> w237
            tunnel: w236 -> [w260 w315 w396 w535 w657 w779 _ w1116]
            tunnel: w235 -> [_ _ _ _ _ _ w876 _]
            frame "Offset" {
              n77 = local read "Offset array"() -> (w265:dbl[])
              n78 = local read "Gain (V/A)"() -> (w269:dbl)
              n79 = local read "DaQ"() -> (w256:bool)
              n80 = Unbundle(w271) -> ("read buffer"=w259:string, "Output"=w255:dbl)  [unwired: 2 out]
              n81 = Divide(x=w269, y=1000000000000.0) -> (x/y=w267:dbl)
              n82 = case shown="False" w256 {
                tunnel: [w279 w280] -> w270
                tunnel: w259 -> [w278 _]
                tunnel: w255 -> [_ w280]
                frame False {
                  n83 = Fract/Exp String To Number(string=w278) -> (number=w279:dbl)  [unwired: 3 in, 1 out]
                }
                frame True {
                }
              }
              n84 = Divide(x=w270, y=w267) -> (x/y=w266:dbl)
              n85 = Build Array (concatenate)(w265, w266) -> (w262:dbl[])
              "Offset array" <- w262
              n86 = Array Size(array=w262) -> (size(s)=w264:i32)
              n87 = Greater?(x=w264, y="Count") -> (0:w263:bool)
              n88 = call-poly <vilib>:"Mean.vi"("X"=w262) -> ("mean"=w258:dbl)  [unwired: 1 out]
              "Dc offset" <- w258
              n89 = case shown="True" w263 {
                tunnel: [Mode."Offset" ("Enum") Mode."Process" ("Enum")] -> w261
                tunnel: w258 -> [_ w288]
                tunnel: [TRUE FALSE] -> w257
                frame False {
                }
                frame True {
                  w284 = 0.0 ("Actual2")
                  n90 = case shown="True" "First Offset?" {
                    tunnel: w288 -> [_ w294]
                    frame False {
                    }
                    frame True {
                      n91 = local read "refnum out"() -> (w300:refnum<file>)
                      n92 = local read "Keithley (IV conv) averaging"() -> (w293:i32)
                      n93 = local read "B/V (T/V)"() -> (w295:dbl)
                      n94 = local read "Gain (V/A)"() -> (w296:dbl)
                      n95 = local write "First Offset?"(FALSE ("First Offset?")) -> ()
                      n96 = local read "Sample area (mm^2)"() -> (w292:dbl)
                      n97 = local read "B0 (T)"() -> (w297:dbl)
                      n98 = local read "I0 (A)"() -> (w298:dbl)
                      n99 = local read "V/I (Ohm)"() -> (w299:dbl)
                      n100 = call "File_header_diag.vi"("Averaging"=w293, "Sample area"=w292, "OFFSET"=w294, "B0"=w297, "B/V"=w295, "I0"=w298, "V/I"=w299, "Gain"=w296, "Byte Stream File in"=w300) -> ()  [unwired: 3 in]
                    }
                  }
                  n101 = local write "Ready2Step"(TRUE ("Ready2Step")) -> ()
                  n102 = local write "Offset?"(TRUE ("Offset?")) -> ()
                  n103 = Get Date/Time In Seconds() -> (seconds since 1Jan1904=→"Start time":timestamp)
                  n104 = local write "Actual2"(w284) -> ()
                  n105 = local write "Last2"(w284) -> ()
                }
              }
            }
            frame "Process", Default {
              # "Converted to pA"
              # "Magnetic Field"
              # "IV converter"
              # "Elapsed Time"
              n106 = local read "DaQ"() -> (w303:bool)
              n107 = local read "Start time"() -> (w337:timestamp)
              n108 = Unbundle(w339) -> ("seconds since 1Jan1904"=w338:timestamp, "read buffer"=w304:string, "read buffer"=w321:string, "Output"=w301:dbl)
              n109 = local read "B/V (T/V)"() -> (w311:dbl)
              n110 = case shown="False" w303 {
                tunnel: w304 -> [w343 _]
                tunnel: [w342 w344] -> w302
                tunnel: w301 -> [_ w344]
                frame False {
                  n111 = Fract/Exp String To Number(string=w343) -> (number=w342:dbl)  [unwired: 3 in, 1 out]
                }
                frame True {
                }
              }
              n112 = Fract/Exp String To Number(string=w321) -> (number=w331:dbl)  [unwired: 3 in, 1 out]
              n113 = Subtract(x=w338, y=w337) -> (x-y=w316:dbl)
              n114 = Divide(x="Gain (V/A)", y=1000000000000.0) -> (x/y=w314:dbl)
              n115 = Divide(x=w302, y=w314) -> (x/y=w309:dbl)
              n116 = Subtract(x=w316, y=w315) -> (x-y=→"Time Lag":dbl)
              n117 = Build Array (concatenate)(w329, w316) -> (w336:dbl[])
              "Elapsed Time (s)" <- w336
              n118 = local read "Dc offset"() -> (w307:dbl)
              n119 = Subtract(x=w309, y=w307) -> (x-y=w308:dbl)
              "Actual Current (pA)" <- w308
              n120 = Build Array (concatenate)(w334, w308) -> (w335:dbl[])
              "Measured Current (pA)" <- w335
              n121 = local read "B0 (T)"() -> (w310:dbl)
              n122 = xnode "B(U) conversion"("V"=w331, "BpV"=w311, "B0"=w310) -> ("Result"=w330:dbl)  [unwired: 1 in, 1 out]
              "Actual B Field (T)" <- w330
              n123 = Build Array (concatenate)(w332, w330) -> (w333:dbl[])
              "Magnetic Field (T)" <- w333
              n124 = Quotient & Remainder(x=w316, y="Temp Refresh (s)") -> (floor(x/y)=w328:dbl)  [unwired: 1 out]
              n125 = Greater?(x=w328, y=w327) -> (0:w326:bool)
              "Read?" <- w326
              n126 = case shown="True" w326 {
                tunnel: [w348 w373] -> w323
                tunnel: w320 -> [w349 w372]
                tunnel: [w349 w352] -> w319
                tunnel: T6 {"Com Port"=1, "ISOBUS Address"=0, "GPIB Address"=25, "Communication"=enum."GPIB"} ("Address") -> [_ w371]
                tunnel: [w347 w367] -> w305
                frame False {
                  n127 = local read "Setpoint Temperature (K)"() -> (w347:dbl)
                  n128 = local read "Actual Temperature (K)"() -> (w348:dbl)
                }
                frame True {
                  w368 = u32 1000 ("byte count")
                  # "Temperature/Magnet read"
                  n129 = local read "Lock_in_Amplifier"() -> (w356:refnum<visa-resource-name>)
                  n130 = local read "Lake Shore"() -> (w370:refnum<visa-resource-name>)
                  n131 = local read "Magnet"() -> (w359:bool)
                  n132 = case shown="False" w359 {
                    tunnel: w371 -> [_ w377]
                    frame False {
                    }
                    frame True {
                      n133 = call "GPIB - BusCommand.vi"("Command"="R7" ("format string"), "Address"=w377) -> ("Reply"=w378:string)  [unwired: 1 out]
                      n134 = Scan From String(format string="R%f" ("remaining string"), input string=w378) -> (output 1=w376:dbl)  [unwired: 3 in, 3 out]
                      n135 = local write "Actual Field (T)"(w376) -> ()
                    }
                  }
                  n136 = VISA Write(VISA resource name=w370, write buffer="KRDG?a", error in (no error)=w372) -> (VISA resource name out=w366:refnum<visa-resource-name>, error out=w364:errorcluster)  [unwired: 1 out]
                  n137 = VISA Read(VISA resource name=w366, byte count=w368, error in (no error)=w364) -> (VISA resource name out=w365:refnum<visa-resource-name>, read buffer=w374:string, error out=w363:errorcluster)  [unwired: 1 out]
                  n138 = VISA Write(VISA resource name=w365, write buffer="SETP?a", error in (no error)=w363) -> (VISA resource name out=w361:refnum<visa-resource-name>, error out=w362:errorcluster)  [unwired: 1 out]
                  n139 = Fract/Exp String To Number(string=w374) -> (number=w373:dbl)  [unwired: 3 in, 1 out]
                  n140 = VISA Read(VISA resource name=w361, byte count=w368, error in (no error)=w362) -> (read buffer=w360:string, error out=w358:errorcluster)  [unwired: 2 out]
                  n141 = VISA Write(VISA resource name=w356, write buffer="OUTP? 3", error in (no error)=w358) -> (VISA resource name out=w355:refnum<visa-resource-name>, error out=w357:errorcluster)  [unwired: 1 out]
                  n142 = VISA Read(VISA resource name=w355, byte count=u32 1000, error in (no error)=w357) -> (read buffer=w351:string, error out=w352:errorcluster)  [unwired: 2 out]
                  n143 = Fract/Exp String To Number(string=w351) -> (number=→"LockInR":dbl)  [unwired: 3 in, 1 out]
                  n144 = Fract/Exp String To Number(string=w360) -> (number=w367:dbl)  [unwired: 3 in, 1 out]
                }
              }
              "Actual Temperature (K)" <- w323
              "Setpoint Temperature (K)" <- w305
              n145 = Build Array (concatenate)(w325, w323) -> (w324:dbl[])
              "Temperature array" <- w324
              n146 = case shown="True" "Sweep" {
                tunnel: [Mode."Plot" ("Enum") Mode."Sweep" ("Enum")] -> w322
                frame False {
                }
                frame True {
                }
              }
            }
            frame "Sweep" {
              n147 = local read "Temp/Magnetic Field"() -> (w394:bool)
              n148 = case shown="False" w394 {
                tunnel: w404 -> [w417 w482]
                tunnel: [w416 w481] -> w403
                frame False {
                  n149 = local read "Stepping Mode"() -> (w411:bool)
                  n150 = local read "Actual Field (T)"() -> (w413:dbl)
                  n151 = local read "Min Field (T)"() -> (w412:dbl)
                  n152 = case shown="True" w411 {
                    tunnel: [w419 w420] -> w410
                    frame False {
                      n153 = local read "Read?"() -> (w419:bool)
                    }
                    frame True {
                      n154 = local read "Ready2Step"() -> (w420:bool)
                    }
                  }
                  n155 = local read "Max Field (T)"() -> (w418:dbl)
                  n156 = Greater Or Equal?(x=w412, y=w413) -> (x >= y?=w415:bool)
                  n157 = Compound Arithmetic op=AND(w415, w410) -> (w414:bool)
                  n158 = case shown="False" w414 {
                    tunnel: [w423 w462] -> w416
                    tunnel: w418 -> [w421 w461]
                    tunnel: w412 -> [_ w460]
                    tunnel: w413 -> [_ w458]
                    tunnel: w417 -> [w424 w457]
                    frame True {
                      # "Ramp Up"
                      n159 = case shown="False" "First?" {
                        tunnel: [TRUE ("Save") FALSE ("Save")] -> w427
                        tunnel: [w449 w453] -> w426
                        frame False {
                          n160 = local read "Counter"() -> (w452:i8)
                          n161 = local write "Actual Polarization"(0.0 ("Actual Polarization")) -> ()
                          n162 = Increment(x=w452) -> (x+1=w449:i8)
                          n163 = local write "Counter"(w449) -> ()
                        }
                        frame True {
                          n164 = local read "Counter"() -> (w453:i8)
                          n165 = local write "First?"(FALSE ("First?")) -> ()
                        }
                      }
                      "Reset" <- w427
                      n166 = local write "Read?"(FALSE ("Read?")) -> ()
                      n167 = local read "Record ALL"() -> (w422:bool)
                      n168 = case shown="False" w422 {
                        tunnel: w426 -> [_ w434]
                        tunnel: [FALSE w432] -> w425
                        frame False {
                        }
                        frame True {
                          n169 = Greater?(x=w434, y="Max Countl") -> (0:w432:bool)
                        }
                      }
                      n170 = case shown="False" w425 {
                        tunnel: w424 -> [w441 w448]
                        tunnel: [w440 w448] -> w423
                        tunnel: w421 -> [w439 _]
                        frame False {
                          n171 = local read "Stepping Mode"() -> (w437:bool)
                          n172 = local read "Magnet"() -> (w438:bool)
                          n173 = Not(x=w437) -> (.not. x?=w436:bool)
                          n174 = And(x=w436, y=w438) -> (x .and. y?=w435:bool)
                          n175 = case shown="False" w435 {
                            tunnel: w441 -> [w442 w445]
                            tunnel: [w442 w444] -> w440
                            tunnel: w439 -> [_ w443]
                            frame False {
                            }
                            frame True {
                              n176 = call "Set_B.vi"("error in (no error)"=w445, "address string"="25", "Set Field (T)"=w443) -> ("error out"=w444:errorcluster)  [unwired: 8 in]
                            }
                          }
                          "Target Field" <- w439
                        }
                        frame True {
                          "New" <- TRUE
                        }
                      }
                      "Up/Down" <- FALSE ("Up/Down")
                    }
                    frame False {
                      n177 = Less Or Equal?(x=w461, y=w458) -> (x <= y?=w459:bool)
                      n178 = case shown="False" w459 {
                        tunnel: [w463 w470] -> w462
                        tunnel: w460 -> [_ w468]
                        tunnel: w457 -> [w463 w471]
                        frame False {
                        }
                        frame True {
                          # "Resetting at the end of every cycle"
                          # "Ramp Dn"
                          n179 = local write "Up/Down"(TRUE ("Up/Down")) -> ()
                          n180 = local read "Stepping Mode"() -> (w467:bool)
                          n181 = local read "Magnet"() -> (w465:bool)
                          n182 = local write "Target Field"(w468) -> ()
                          n183 = Not(x=w467) -> (.not. x?=w466:bool)
                          n184 = And(x=w465, y=w466) -> (x .and. y?=w464:bool)
                          n185 = local write "Reset"(TRUE ("Reset")) -> ()
                          n186 = case shown="True" w464 {
                            tunnel: w471 -> [w473 w476]
                            tunnel: [w473 w475] -> w470
                            tunnel: w468 -> [_ w474]
                            frame False {
                            }
                            frame True {
                              n187 = call "Set_B.vi"("error in (no error)"=w476, "address string"="25", "Set Field (T)"=w474) -> ("error out"=w475:errorcluster)  [unwired: 8 in]
                            }
                          }
                        }
                      }
                      n188 = local write "Read?"(FALSE ("Read?")) -> ()
                    }
                  }
                }
                frame True {
                  n189 = local read "Setpoint Temperature (K)"() -> (w480:dbl)
                  n190 = local read "Min Temperature (K)"() -> (w479:dbl)
                  n191 = local read "Read?"() -> (w485:bool)
                  n192 = local read "Max temperature (K)"() -> (w478:dbl)
                  n193 = Equal?(x=w480, y=w479) -> (x = y?=w483:bool)
                  n194 = And(x=w483, y=w485) -> (x .and. y?=w484:bool)
                  n195 = case shown="False" w484 {
                    tunnel: [w487 w523] -> w481
                    tunnel: w478 -> [w494 w522]
                    tunnel: w479 -> [_ w521]
                    tunnel: w480 -> [_ w519]
                    tunnel: w482 -> [w488 w518]
                    frame True {
                      # "Ramp Up"
                      n196 = local read "First?"() -> (w498:bool)
                      n197 = case shown="False" w498 {
                        tunnel: [TRUE ("Save") FALSE ("Save")] -> w490
                        tunnel: [w510 w516] -> w492
                        frame False {
                          n198 = local read "Counter"() -> (w513:i8)
                          n199 = local write "Actual Polarization"(0.0 ("Actual Polarization")) -> ()
                          n200 = Increment(x=w513) -> (x+1=w510:i8)
                          n201 = local write "Counter"(w510) -> ()
                        }
                        frame True {
                          n202 = local read "Counter"() -> (w516:i8)
                          n203 = local write "First?"(FALSE ("First?")) -> ()
                        }
                      }
                      n204 = local write "Read?"(FALSE ("Read?")) -> ()
                      n205 = local write "Up/Down"(FALSE ("Up/Down")) -> ()
                      n206 = Number To Fractional String(number=w494, precision (6)=i16 3) -> (F-format string=w496:string)  [unwired: 2 in]
                      n207 = local read "Record ALL"() -> (w493:bool)
                      n208 = Concatenate Strings("SETP 1," ("write buffer"), w496) -> (w489:string)
                      n209 = case shown="True" w493 {
                        tunnel: w492 -> [_ w509]
                        tunnel: [FALSE w508] -> w491
                        frame False {
                        }
                        frame True {
                          n210 = local read "Max Countl"() -> (w507:i32)
                          n211 = Greater?(x=w509, y=w507) -> (0:w508:bool)
                        }
                      }
                      n212 = local write "Reset"(w490) -> ()
                      n213 = case shown="True" w491 {
                        tunnel: w489 -> [w503 _]
                        tunnel: w488 -> [w501 w504]
                        tunnel: [w500 w504] -> w487
                        frame False {
                          n214 = local read "Lake Shore"() -> (w502:refnum<visa-resource-name>)
                          n215 = VISA Write(VISA resource name=w502, write buffer=w503, error in (no error)=w501) -> (error out=w500:errorcluster)  [unwired: 2 out]
                        }
                        frame True {
                          n216 = local write "New"(TRUE ("New")) -> ()
                        }
                      }
                    }
                    frame False {
                      n217 = Equal?(x=w522, y=w519) -> (x = y?=w520:bool)
                      n218 = case shown="True" w520 {
                        tunnel: [w524 w528] -> w523
                        tunnel: w521 -> [_ w527]
                        tunnel: w518 -> [w524 w529]
                        frame False {
                        }
                        frame True {
                          w525 = TRUE ("Reset")
                          # "Ramp Dn"
                          n219 = Number To Fractional String(number=w527, precision (6)=i16 3) -> (F-format string=w531:string)  [unwired: 2 in]
                          n220 = local write "Reset"(w525) -> ()
                          n221 = local write "Up/Down"(w525) -> ()
                          n222 = local read "Lake Shore"() -> (w526:refnum<visa-resource-name>)
                          n223 = Concatenate Strings("SETP 1," ("write buffer"), w531) -> (w533:string)
                          n224 = VISA Write(VISA resource name=w526, write buffer=w533, error in (no error)=w529) -> (error out=w528:errorcluster)  [unwired: 2 out]
                        }
                      }
                      n225 = local write "Read?"(FALSE ("Read?")) -> ()
                    }
                  }
                }
              }
              n226 = local read "Magnet"() -> (w393:bool)
              n227 = case shown="True" w393 {
                tunnel: [Mode."StepDelta" ("Enum") w407] -> w395
                frame False {
                }
                frame True {
                  n228 = local read "Stepping Mode"() -> (w406:bool)
                  n229 = case shown="False" w406 {
                    tunnel: [Mode."Plot" ("Enum") Mode."StepDelta" ("Enum")] -> w407
                    frame False {
                    }
                    frame True {
                    }
                  }
                }
              }
            }
            frame "StepDelta" {
              n230 = local read "Stepping Mode"() -> (w536:bool)
              n231 = case shown="True" w536 {
                tunnel: w538 -> [w547 w602]
                tunnel: [w546 w599] -> w537
                tunnel: w535 -> [_ w601]
                tunnel: [w545 w600] -> w534
                frame False {
                  n232 = flat-sequence {
                    tunnel: w547 -> [w556]
                    tunnel: [w555] -> w546
                    tunnel: [Mode."Plot" ("Enum")] -> w545
                    frame #0 {
                      # "Check if it is time to step Field"
                      n233 = local read "Sweep Rate (T/min)"() -> (w557:dbl)
                      n234 = local read "B/V (T/V)"() -> (w549:dbl)
                      n235 = local read "Time Lag"() -> (w553:dbl)
                      n236 = xnode "Sweep Delay"("SweepRate"=w557, "Resolution"=0.001 ("Voltage Step (V)"), "BpV"=w549) -> ("Result"=w554:dbl)  [unwired: 1 in, 1 out]
                      n237 = Divide(x=w553, y=w554) -> (x/y=w551:dbl)
                      n238 = Multiply(x=0.001 ("y"), y=w551) -> (x*y=w550:dbl)
                      "deltaUaux" <- w550
                      n239 = stacked-sequence {
                        tunnel: w556 -> [_ w581]
                        tunnel: [_ w580] -> w555
                        tunnel: w550 -> [w559 _]
                        frame #0 {
                          n240 = local read "Actual Voltage (V)"() -> (w564:dbl)
                          n241 = local read "Up/Down"() -> (w565:bool)
                          n242 = Add(x=w564, y=w559) -> (x+y=w561:dbl)
                          n243 = Subtract(x=w564, y=w559) -> (x-y=w560:dbl)
                          n244 = Select(t=w560, s=w565, f=w561) -> (s? t:f=w563:dbl)
                          "Actual Voltage (V)" <- w563
                          n245 = local read "V/I (Ohm)"() -> (w566:dbl)
                          n246 = local read "B/V (T/V)"() -> (w567:dbl)
                          n247 = xnode "AUXtoB"("BpV"=w567, "Rm"=w566, "Aux"=w563) -> ("Result"=w562:dbl)  [unwired: 1 in, 1 out]
                          n248 = local write "Actual Field (T)"(w562) -> ()
                        }
                        frame #1 {
                          n249 = local read "Actual Voltage (V)"() -> (w586:dbl)
                          n250 = local read "Lock_in_Amplifier"() -> (w582:refnum<visa-resource-name>)
                          n251 = Format Into String(w586) -> (resulting string=w585:string)  [unwired: 3 in, 1 out]
                          n252 = Concatenate Strings("AUXV 1,", w585) -> (w583:string)
                          n253 = VISA Write(VISA resource name=w582, write buffer=w583, error in (no error)=w581) -> (error out=w580:errorcluster)  [unwired: 2 out]
                        }
                      }
                    }
                  }
                }
                frame True {
                  n254 = local read "Up/Down"() -> (w603:bool)
                  n255 = local read "Actual Field (T)"() -> (w604:dbl)
                  n256 = stacked-sequence {
                    tunnel: "Field Step (T)" -> [w610 _]
                    tunnel: w604 -> [w609 _]
                    tunnel: w603 -> [w608 _]
                    tunnel: w602 -> [w607 w623]
                    tunnel: [_ w628] -> _
                    tunnel: w601 -> [_ w628]
                    tunnel: [_ w624] -> w600
                    tunnel: [_ w623] -> w599
                    frame #0 {
                      n257 = local read "Ready2Step"() -> (w606:bool)
                      n258 = case shown="True" w606 {
                        tunnel: w610 -> [_ w616]
                        tunnel: w609 -> [_ w617]
                        tunnel: w608 -> [_ w615]
                        tunnel: w607 -> [w611 w614]
                        tunnel: [w611 w613] -> _
                        frame False {
                        }
                        frame True {
                          n259 = Add(x=w617, y=w616) -> (x+y=w619:dbl)
                          n260 = Subtract(x=w617, y=w616) -> (x-y=w618:dbl)
                          n261 = Select(t=w618, s=w615, f=w619) -> (s? t:f=w621:dbl)
                          n262 = call "Set_B.vi"("error in (no error)"=w614, "address string"="25", "Set Field (T)"=w621) -> ("error out"=w613:errorcluster)  [unwired: 8 in]
                          n263 = local write "Ready2Step"(FALSE ("Ready2Step")) -> ()
                        }
                      }
                    }
                    frame #1 {
                      n264 = local read "Last2"() -> (w626:dbl)
                      n265 = Quotient & Remainder(x=w628, y="Window (s)") -> (floor(x/y)=w622:dbl)  [unwired: 1 out]
                      "Actual2" <- w622
                      n266 = Greater?(x=w622, y=w626) -> (0:w625:bool)
                      n267 = case shown="True" w625 {
                        tunnel: w622 -> [_ w635]
                        tunnel: [Mode."Plot" ("Enum") w633] -> w624
                        frame False {
                          n268 = local read "Actual Current (pA)"() -> (→"I(t)":dbl)
                          n269 = local read "Actual B Field (T)"() -> (→"B(t)":dbl)
                          n270 = local read "Actual Polarization"() -> (→"P(t)":dbl)
                        }
                        frame True {
                          n271 = case shown="True" "ReOffset" {
                            tunnel: [Mode."Plot" ("Enum") Mode."Offset" ("Enum")] -> w633
                            frame False {
                              "Ready2Step" <- TRUE ("Ready2Step 2")
                            }
                            frame True {
                              n272 = local read "Sampling rate (Hz)"() -> (w639:dbl)
                              n273 = local write "Offset array"(dbl[] []) -> ()
                              n274 = local write "Offset?"(FALSE ("Offset?")) -> ()
                              n275 = Reciprocal(x=w639) -> (1/x=w638:dbl)
                              n276 = Divide(x="Dwell Time (s)", y=w638) -> (x/y=w642:dbl)
                              n277 = local write "Count"(w642) -> ()
                            }
                          }
                          "Last2" <- w635
                        }
                      }
                    }
                  }
                }
              }
            }
            frame "Plot" {
              # "dI"
              n278 = local read "P(uC/mm^2)"() -> (w646:dbl[])
              n279 = local read "Actual Polarization"() -> (w645:dbl)
              n280 = local read "Actual Current (pA)"() -> (w647:dbl)
              n281 = local read "Time Lag"() -> (w659:dbl)
              n282 = Multiply(x=w647, y=w659) -> (x*y=w651:dbl)
              n283 = Divide(x=w651, y="Sample area (mm^2)") -> (x/y=w650:dbl)
              n284 = Add(x=w650, y=w645) -> (x+y=w649:dbl)
              "Actual Polarization" <- w649
              n285 = local read "Temp/Magnetic Field"() -> (w660:bool)
              n286 = Build Array (concatenate)(w646, w649) -> (→"P(uC/mm^2)":dbl[])
              n287 = case shown="True" w660 {
                tunnel: w657 -> [_ w711]
                tunnel: w654 -> [_ w707]
                tunnel: w649 -> [w667 w708]
                frame False {
                  # "Magnetic Field plotting"
                  n288 = local read "Up/Down"() -> (w672:bool)
                  n289 = case shown="True" w672 {
                    frame True {
                      # "Down"
                      n290 = local read "I(B) 3"() -> (w682:cluster{dbl[], dbl[]}[])
                      n291 = local read "I(B) 3"() -> (w686:cluster{dbl[], dbl[]}[])
                      n292 = Index Array(array=w682, index=1) -> (element=w680:cluster{dbl[], dbl[]})
                      n293 = Unbundle(w680) -> (w679:dbl[], w678:dbl[])
                      n294 = Index Array(array=w686, index=i8 0 ("t")) -> (element=w683:cluster{dbl[], dbl[]})
                      n295 = local read "Actual Current (pA)"() -> (w673:dbl)
                      n296 = local read "Actual B Field (T)"() -> (w675:dbl)
                      n297 = Build Array (concatenate)(w679, w675) -> (w677:dbl[])
                      n298 = Build Array (concatenate)(w678, w673) -> (w676:dbl[])
                      n299 = Bundle(w677, w676) -> (w674:cluster{dbl[], dbl[]})  [unwired: 1 in]
                      n300 = Build Array(w683, w674) -> (w684:cluster{dbl[], dbl[]}[])
                      n301 = local write "I(B) 3"(w684) -> ()
                    }
                    frame False {
                      # "Up"
                      n302 = local read "I(B) 3"() -> (w698:cluster{dbl[], dbl[]}[])
                      n303 = local read "I(B) 3"() -> (w700:cluster{dbl[], dbl[]}[])
                      n304 = Index Array(array=w698, index=0) -> (element=w696:cluster{dbl[], dbl[]})
                      n305 = Unbundle(w696) -> (w695:dbl[], w694:dbl[])
                      n306 = Index Array(array=w700, index=i8 1 ("t")) -> (element=w689:cluster{dbl[], dbl[]})
                      n307 = local read "Actual B Field (T)"() -> (w690:dbl)
                      n308 = Build Array (concatenate)(w695, w690) -> (w693:dbl[])
                      n309 = local read "Actual Current (pA)"() -> (w687:dbl)
                      n310 = Build Array (concatenate)(w694, w687) -> (w692:dbl[])
                      n311 = Bundle(w693, w692) -> (w691:cluster{dbl[], dbl[]})  [unwired: 1 in]
                      n312 = Build Array(w691, w689) -> (w688:cluster{dbl[], dbl[]}[])
                      n313 = local write "I(B) 3"(w688) -> ()
                    }
                  }
                  n314 = local read "Actual B Field (T)"() -> (w669:dbl)
                  n315 = local read "P(B)"() -> (w671:cluster{"yi":dbl[], dbl[]})
                  n316 = Unbundle(w671) -> ("yi"=w670:dbl[], w668:dbl[])
                  n317 = Build Array (concatenate)(w670, w669) -> (w666:dbl[])
                  n318 = Build Array (concatenate)(w668, w667) -> (w665:dbl[])
                  n319 = Bundle(w666, w665) -> (→"P(B)":cluster{dbl[], dbl[]})  [unwired: 1 in]
                }
                frame True {
                  # "Temperature plotting"
                  n320 = local read "Actual Current (pA)"() -> (w710:dbl)
                  n321 = local read "Actual Temperature (K)"() -> (w709:dbl)
                  n322 = local read "Up/Down"() -> (w703:bool)
                  n323 = local read "P(T)"() -> (w704:cluster{dbl[], dbl[]}[])
                  n324 = local read "Sweep"() -> (w706:bool)
                  n325 = local read "I(T)"() -> (w705:cluster{dbl[], dbl[]}[])
                  n326 = case shown="False" w703 {
                    tunnel: w710 -> [w732 w757]
                    tunnel: w709 -> [w728 w753]
                    tunnel: w708 -> [w726 w751]
                    tunnel: w705 -> [w721 w746]
                    tunnel: w704 -> [w716 w743]
                    tunnel: [w717 w744] -> w702
                    tunnel: [w712 w741] -> w701
                    frame True {
                      n327 = Index Array(array=w721, index=1) -> (element=w725:cluster{dbl[], dbl[]})
                      n328 = Index Array(array=w716, index=1) -> (element=w724:cluster{dbl[], dbl[]})
                      n329 = Index Array(array=w716, index=0) -> (element=w713:cluster{dbl[], dbl[]})
                      n330 = Index Array(array=w721, index=0) -> (element=w718:cluster{dbl[], dbl[]})
                      n331 = Unbundle(w724) -> (w729:dbl[], w727:dbl[])
                      n332 = Unbundle(w725) -> (w736:dbl[], w735:dbl[])
                      n333 = Build Array (concatenate)(w729, w728) -> (w730:dbl[])
                      n334 = Build Array (concatenate)(w727, w726) -> (w731:dbl[])
                      n335 = Build Array (concatenate)(w736, w728) -> (w734:dbl[])
                      n336 = Build Array (concatenate)(w735, w732) -> (w733:dbl[])
                      n337 = Bundle(w730, w731) -> (w714:cluster{dbl[], dbl[]})  [unwired: 1 in]
                      n338 = Bundle(w734, w733) -> (w719:cluster{dbl[], dbl[]})  [unwired: 1 in]
                      n339 = Build Array(w713, w714) -> (w712:cluster{dbl[], dbl[]}[])
                      n340 = Build Array(w718, w719) -> (w717:cluster{dbl[], dbl[]}[])
                    }
                    frame False {
                      n341 = Index Array(array=w746, index=0) -> (element=w750:cluster{dbl[], dbl[]})
                      n342 = Index Array(array=w743, index=0) -> (element=w749:cluster{dbl[], dbl[]})
                      n343 = Index Array(array=w743, index=1) -> (element=w737:cluster{dbl[], dbl[]})
                      n344 = Index Array(array=w746, index=1) -> (element=w740:cluster{dbl[], dbl[]})
                      n345 = Unbundle(w749) -> (w754:dbl[], w752:dbl[])
                      n346 = Unbundle(w750) -> (w761:dbl[], w760:dbl[])
                      n347 = Build Array (concatenate)(w754, w753) -> (w755:dbl[])
                      n348 = Build Array (concatenate)(w752, w751) -> (w756:dbl[])
                      n349 = Build Array (concatenate)(w761, w753) -> (w759:dbl[])
                      n350 = Build Array (concatenate)(w760, w757) -> (w758:dbl[])
                      n351 = Bundle(w755, w756) -> (w738:cluster{dbl[], dbl[]})  [unwired: 1 in]
                      n352 = Bundle(w759, w758) -> (w739:cluster{dbl[], dbl[]})  [unwired: 1 in]
                      n353 = Build Array(w738, w737) -> (w741:cluster{dbl[], dbl[]}[])
                      n354 = Build Array(w739, w740) -> (w744:cluster{dbl[], dbl[]}[])
                    }
                  }
                  "I(T)" <- w702
                  "P(T)" <- w701
                  n355 = case shown="False" w706 {
                    tunnel: w711 -> [w766 _]
                    tunnel: w707 -> [w763 _]
                    frame False {
                      n356 = Quotient & Remainder(x=w766, y="Save Period") -> (x-y*floor(x/y)=w762:dbl)  [unwired: 1 out]
                      n357 = Greater?(x=w763, y=w762) -> (0:w764:bool)
                      n358 = case shown="True" w764 {
                        frame False {
                        }
                        frame True {
                          n359 = local write "Reset"(TRUE) -> ()
                        }
                      }
                    }
                    frame True {
                    }
                  }
                }
              }
            }
            frame "Save" {
              n360 = local read "Reset"() -> (w768:bool)
              n361 = case shown="True" w768 {
                tunnel: w773 -> [w790 w792]
                tunnel: [w790 w795] -> w778
                tunnel: w772 -> [w789 w793]
                tunnel: [w789 w795] -> w777
                tunnel: w774 -> [w788 w794]
                tunnel: [w788 w795] -> w776
                tunnel: [w787 w795] -> w775
                tunnel: w771 -> [w787 w791]
                frame False {
                }
                frame True {
                  n362 = stacked-sequence {
                    tunnel: [_ _ w875] -> w795
                    tunnel: w794 -> [_ w870 _]
                    tunnel: w793 -> [w798 w868 _]
                    tunnel: w792 -> [w799 w869 _]
                    tunnel: w791 -> [w797 w866 _]
                    frame #0 {
                      n363 = local read "Temp/Magnetic Field"() -> (w796:bool)
                      n364 = case shown="False" w796 {
                        tunnel: w799 -> [w826 w853]
                        tunnel: w798 -> [w825 w852]
                        tunnel: w797 -> [w816 w843]
                        frame False {
                          n365 = local read "B array"() -> (w810:dbl[])
                          n366 = local read "Counter"() -> (w824:i8)
                          n367 = local read "Averaged I(B)"() -> (w801:dbl[][])
                          n368 = local read "Up/Down"() -> (w827:bool)
                          n369 = local read "Sample area (mm^2)"() -> (w806:dbl)
                          n370 = call "Average_IBP_curves_baseline.vi"("I in"=w825, "Averaged P(B) In"="Averaged P(B)", "Counter"=w824, "B0"="Threshold B (T)", "Averaged I(B) In"=w801, "t in"=w816, "B in"=w826, "Averaged dt in"="Averaged dt", "Up/Down"=w827, "Sample area(mm^2)"=w806, "B array"=w810) -> ("Averaged dt Out"=w813:dbl[][], "Averaged P(B) Out"=w802:dbl[][], "BaselineSubtracted I(B)"=w800:dbl[][])  [unwired: 1 in, 1 out]
                          "Averaged I(B)" <- w800
                          n371 = Index Array(array=w802, index (row)=0 ("disabled index (col)")) -> (element=w811:dbl[])  [unwired: 1 in]
                          n372 = Index Array(array=w802, index (row)=1 ("disabled index (col)")) -> (element=w812:dbl[])  [unwired: 1 in]
                          n373 = Index Array(array=w800, index (row)=0 ("disabled index (col)")) -> (element=w818:dbl[])  [unwired: 1 in]
                          n374 = Index Array(array=w800, index (row)=1 ("disabled index (col)")) -> (element=w817:dbl[])  [unwired: 1 in]
                          n375 = local write "Averaged dt"(w813) -> ()
                          n376 = Bundle("B array"=w810, "Averaged P(B) Out"=w811) -> (w809:T7)  [unwired: 1 in]
                          n377 = Bundle("B array"=w810, "Averaged P(B) Out"=w812) -> (w808:T7)  [unwired: 1 in]
                          n378 = local write "Averaged P(B)"(w802) -> ()
                          n379 = Bundle("B array"=w810, "BaselineSubtracted I(B)"=w818) -> (w823:T8)  [unwired: 1 in]
                          n380 = Bundle("B array"=w810, "BaselineSubtracted I(B)"=w817) -> (w822:T8)  [unwired: 1 in]
                          n381 = Build Array(w809, w808) -> (→"P(B) /Averaged/":T9)
                          n382 = Build Array(w823, w822) -> (→"I(B) /Averaged/":T10)
                        }
                        frame True {
                          n383 = local read "T array"() -> (w838:dbl[])
                          n384 = local read "Counter"() -> (w851:i8)
                          n385 = local read "Averaged I(T)"() -> (w830:dbl[][])
                          n386 = local read "Up/Down"() -> (w854:bool)
                          n387 = local read "Averaged dt"() -> (w829:dbl[][])
                          n388 = local read "Sample area (mm^2)"() -> (w834:dbl)
                          n389 = call "Average_ITP_curves.vi"("I in"=w852, "Averaged P(T) In"="Averaged P(T)", "Counter"=w851, "Averaged I(T) In"=w830, "t in"=w843, "T in"=w853, "Averaged dt in"=w829, "Up/Down"=w854, "Sample area(mm^2)"=w834, "T array"=w838) -> ("Averaged I(B) out"=w828:dbl[][], "Averaged dt Out"=w841:dbl[][], "Averaged P(T) Out"=w831:dbl[][])  [unwired: 3 in]
                          "Averaged I(T)" <- w828
                          n390 = Index Array(array=w831, index (row)=0 ("disabled index (col)")) -> (element=w839:dbl[])  [unwired: 1 in]
                          n391 = Index Array(array=w831, index (row)=1 ("disabled index (col)")) -> (element=w840:dbl[])  [unwired: 1 in]
                          n392 = Index Array(array=w828, index (row)=0 ("disabled index (col)")) -> (element=w845:dbl[])  [unwired: 1 in]
                          n393 = Index Array(array=w828, index (row)=1 ("disabled index (col)")) -> (element=w844:dbl[])  [unwired: 1 in]
                          n394 = local write "Averaged dt"(w841) -> ()
                          n395 = Bundle("T array"=w838, "Averaged P(T) Out"=w839) -> (w837:T11)  [unwired: 1 in]
                          n396 = Bundle("T array"=w838, "Averaged P(T) Out"=w840) -> (w836:T11)  [unwired: 1 in]
                          n397 = local write "Averaged P(T)"(w831) -> ()
                          n398 = Bundle("T array"=w838, "Averaged I(B) out"=w845) -> (w850:T12)  [unwired: 1 in]
                          n399 = Bundle("T array"=w838, "Averaged I(B) out"=w844) -> (w849:T12)  [unwired: 1 in]
                          n400 = Build Array(w837, w836) -> (→"P(T) /Averaged/":T13)
                          n401 = Build Array(w850, w849) -> (→"I(T) /Averaged/":T14)
                        }
                      }
                    }
                    frame #1 {
                      # "Save and Reset"
                      n402 = local read "Up/Down"() -> (w856:bool)
                      n403 = local read "Measurement File"() -> (w861:path)
                      n404 = local read "P(uC/mm^2)"() -> (w867:dbl[])
                      n405 = case shown="True" w856 {
                        tunnel: [w872 w873] -> w855
                        frame False {
                          n406 = local read "Measurement File_dn"() -> (w872:path)
                        }
                        frame True {
                          n407 = local read "Measurement File_up"() -> (w873:path)
                        }
                      }
                      n408 = Build Array(w870, w869, w868, w866, w867) -> (w860:dbl[][])
                      n409 = case shown="True" "Reset IB?" {
                        frame False {
                        }
                        frame True {
                          n410 = local read "Up/Down"() -> (w874:bool)
                          n411 = case shown="False" w874 {
                            frame False {
                              n412 = invoke on="I(B) 3" class="XYGraph (strict)" method="Reinit To Default"() -> ()  [unwired: 3 in, 3 out]
                              n413 = invoke on="I(T)" class="XYGraph (strict)" method="Reinit To Default"() -> ()  [unwired: 3 in, 3 out]
                            }
                            frame True {
                            }
                          }
                        }
                      }
                      n414 = call-poly <vilib>:"Write Delimited Spreadsheet.vi"("file path (dialog if empty)"=w861, "format (%.3f)"="%.5g", "2D data"=w860, "append to file? (F)"=TRUE, "transpose? (F)"=TRUE) -> ()  [unwired: 9 in, 2 out]
                      n415 = call-poly <vilib>:"Write Delimited Spreadsheet.vi"("file path (dialog if empty)"=w855, "format (%.3f)"="%.5g", "2D data"=w860, "append to file? (F)"=TRUE ("transpose? (F)"), "transpose? (F)"=FALSE ("append to file? (F)")) -> ()  [unwired: 9 in, 2 out]
                      n416 = local write "Reset"(FALSE ("Save")) -> ()
                    }
                    frame #2 {
                      w875 = dbl[] []
                      n417 = local write "P(uC/mm^2)"(w875) -> ()
                    }
                  }
                }
              }
              n418 = local read "New"() -> (w770:bool)
              n419 = case shown="False" w770 {
                tunnel: [Mode."Return" ("Enum") Mode."New" ("Enum")] -> w782
                tunnel: [TRUE FALSE] -> w769
                frame False {
                }
                frame True {
                }
              }
            }
            frame "New" {
              n420 = stacked-sequence {
                seq-local: [_ _ _ _ w1023 _ _] -> [_ _ _ _ _ w1040 _]
                seq-local: [_ _ w960 _ _ _ _] -> [_ _ _ w996 _ _ _]
                seq-local: [_ _ _ w995 _ _ _] -> [_ _ _ _ w1021 _ _]
                seq-local: [_ w915 _ _ _ _ _] -> [_ _ w954 _ _ _ _]
                tunnel: T6 {"Com Port"=1, "ISOBUS Address"=0, "GPIB Address"=25, "Communication"=enum."GPIB"} ("Address") -> [_ _ w959 w1001 _ _ _]
                tunnel: w878 -> [_ w916 _ _ _ w1041 _]
                tunnel: [_ _ _ _ _ w1043 _] -> w877
                tunnel: w876 -> [_ w919 _ _ _ _ _]
                frame #0 {
                  w905 = 1 ("index (row)")
                  w904 = 0 ("index (row)")
                  # "Save averages"
                  n421 = local read "Temp/Magnetic Field"() -> (w888:bool)
                  n422 = case shown="True" w888 {
                    tunnel: [w912 w913] -> w903
                    tunnel: [w911 w914] -> w893
                    frame False {
                      n423 = local read "Averaged P(B)"() -> (w912:dbl[][])
                      n424 = local read "I(B) /Averaged/"() -> (w911:cluster{"B array":dbl[], dbl[]}[])
                    }
                    frame True {
                      n425 = local read "Averaged P(T)"() -> (w913:dbl[][])
                      n426 = local read "I(T) /Averaged/"() -> (w914:cluster{"B array":dbl[], dbl[]}[])
                    }
                  }
                  n427 = local read "Measurement File_average"() -> (w892:path)
                  n428 = local read "Averaged dt"() -> (w901:dbl[][])
                  n429 = Index Array(array=w901, index (row)=w904) -> (element=w902:dbl[])  [unwired: 1 in]
                  n430 = Index Array(array=w901, index (row)=w905) -> (element=w909:dbl[])  [unwired: 1 in]
                  n431 = Index Array(array=w893, index=1) -> (element=w897:cluster{"B array":dbl[], dbl[]})
                  n432 = Index Array(array=w893, index=0) -> (element=w896:cluster{"B array":dbl[], dbl[]})
                  n433 = Unbundle(w897) -> ("B array"=w907:dbl[], w908:dbl[])
                  n434 = Unbundle(w896) -> ("B array"=w898:dbl[], w899:dbl[])
                  n435 = Index Array(array=w903, index (row)=w904) -> (element=w906:dbl[])  [unwired: 1 in]
                  n436 = Index Array(array=w903, index (row)=w905) -> (element=w910:dbl[])  [unwired: 1 in]
                  n437 = Build Array(w898, w899, w902, w906, w907, w908, w909, w910) -> (w900:dbl[][])
                  n438 = call-poly <vilib>:"Write Delimited Spreadsheet.vi"("file path (dialog if empty)"=w892, "format (%.3f)"="%.5g", "2D data"=w900, "append to file? (F)"=TRUE ("transpose? (F)"), "transpose? (F)"=TRUE ("append to file? (F)")) -> ()  [unwired: 9 in, 2 out]
                }
                frame #1 {
                  w927 = dbl[] []
                  # "Reset Flags"
                  n439 = Get Date/Time In Seconds() -> (seconds since 1Jan1904=w928:timestamp)
                  n440 = local write "Measuring"(FALSE ("Measuring")) -> ()
                  n441 = local write "Up/Down"(TRUE ("Up/Down")) -> ()
                  n442 = local write "First?"(TRUE ("First?")) -> ()
                  n443 = local write "Offset?"(FALSE ("Offset?")) -> ()
                  n444 = local write "New"(FALSE ("New")) -> ()
                  n445 = local write "P(uC/mm^2)"(w927) -> ()
                  n446 = local write "Start time"(w928) -> ()
                  n447 = local write "Offset array"(w927) -> ()
                  n448 = local write "Actual Polarization"(0.0 ("Actual Polarization")) -> ()
                  n449 = local write "Up/Down"(TRUE ("Up/Down")) -> ()
                  n450 = local read "Temp/Magnetic Field"() -> (w917:bool)
                  n451 = local write "Reset"(FALSE ("Reset")) -> ()
                  n452 = case shown="False" w917 {
                    tunnel: w916 -> [w933 w946]
                    tunnel: [w931 w946] -> w915
                    frame True {
                      w939 = dbl[] []
                      n453 = local read "B array"() -> (w941:dbl[])
                      n454 = invoke on="I(T)" class="XYGraph (strict)" method="Reinit To Default"() -> ()  [unwired: 3 in, 3 out]
                      n455 = Build Array(w939, w939) -> (w945:dbl[][])
                      n456 = Multiply(x=w941, y=0.0) -> (x*y=w942:dbl[])
                      n457 = Bundle("B array"=w941, w942) -> (w943:cluster{"B array":dbl[], dbl[]})  [unwired: 1 in]
                      n458 = local write "Averaged I(T)"(w945) -> ()
                      n459 = invoke on="P(T)" class="XYGraph (strict)" method="Reinit To Default"() -> ()  [unwired: 3 in, 3 out]
                      n460 = Build Array(w943, w943) -> (w944:cluster{"B array":dbl[], dbl[]}[])
                      n461 = local write "I(T) /Averaged/"(w944) -> ()
                      n462 = local read "Set temperature (K)"() -> (w938:dbl)
                      n463 = Number To Fractional String(number=w938, precision (6)=i16 3) -> (F-format string=w935:string)  [unwired: 2 in]
                      n464 = local read "Lake Shore"() -> (w932:refnum<visa-resource-name>)
                      n465 = Concatenate Strings("SETP 1," ("write buffer"), w935) -> (w937:string)
                      n466 = VISA Write(VISA resource name=w932, write buffer=w937, error in (no error)=w933) -> (error out=w931:errorcluster)  [unwired: 2 out]
                    }
                    frame False {
                      w947 = dbl[] []
                      n467 = local read "B array"() -> (w949:dbl[])
                      n468 = invoke on="I(B) 3" class="XYGraph (strict)" method="Reinit To Default"() -> ()  [unwired: 3 in, 3 out]
                      n469 = Build Array(w947, w947) -> (w953:dbl[][])
                      n470 = Multiply(x=w949, y=0.0) -> (x*y=w950:dbl[])
                      n471 = Bundle("B array"=w949, w950) -> (w951:cluster{"B array":dbl[], dbl[]})  [unwired: 1 in]
                      n472 = local write "Averaged I(B)"(w953) -> ()
                      n473 = invoke on="P(B)" class="XYGraph (strict)" method="Reinit To Default"() -> ()  [unwired: 3 in, 3 out]
                      n474 = Build Array(w951, w951) -> (w952:cluster{"B array":dbl[], dbl[]}[])
                      n475 = local write "I(B) /Averaged/"(w952) -> ()
                    }
                  }
                  n476 = local write "Counter"(i8 0 ("Counter")) -> ()
                  n477 = Flush Queue(queue=w919) -> (remaining elements=→"remaining elements 2":T1)  [unwired: 1 in, 2 out]
                }
                frame #2 {
                  # "Step"
                  n478 = local read "Sweep Rate Array"() -> (w957:dbl[])
                  n479 = local read "T Sweep Rate Array"() -> (w958:dbl[])
                  n480 = local read "Temp/Magnetic Field"() -> (w955:bool)
                  n481 = local read "j"() -> (w964:i32)
                  n482 = Increment(x=w964) -> (x+1=w961:i32)
                  n483 = Select(t=w958, s=w955, f=w957) -> (s? t:f=w956:dbl[])
                  n484 = Array Size(array=w956) -> (size(s)=w963:i32)
                  n485 = Less?(x=w961, y=w963) -> (x < y?=w962:bool)
                  "Step Rate" <- w962
                  n486 = case shown="False" w962 {
                    tunnel: w961 -> [_ w994]
                    tunnel: w954 -> [w971 w993]
                    tunnel: [w970 w993] -> w960
                    tunnel: w959 -> [w969 _]
                    tunnel: w955 -> [w967 _]
                    frame False {
                      # "Step Temp?"
                      n487 = local read "Magnetic Field array (T)"() -> (w966:dbl[])
                      n488 = local read "Temperature Array"() -> (w968:dbl[])
                      n489 = local read "i"() -> (w975:i32)
                      n490 = Select(t=w966, s=w967, f=w968) -> (s? t:f=w965:dbl[])
                      n491 = Increment(x=w975) -> (x+1=w973:i32)
                      n492 = local write "j"(0 ("f")) -> ()
                      n493 = Array Size(array=w965) -> (size(s)=w974:i32)
                      n494 = Less?(x=w973, y=w974) -> (x < y?=w972:bool)
                      "Step Temp" <- w972
                      n495 = case shown="True" w972 {
                        tunnel: w973 -> [_ w992]
                        tunnel: w971 -> [w980 w991]
                        tunnel: [w979 w991] -> w970
                        tunnel: w969 -> [w978 _]
                        frame False {
                          # "Heater OFF"
                          # "Finished"
                          n496 = local write "i"(0 ("i")) -> ()
                          n497 = stacked-sequence {
                            tunnel: w980 -> [w984 _ _]
                            tunnel: [w983 _ _] -> w979
                            tunnel: w978 -> [_ w988 w989]
                            frame #0 {
                              n498 = local read "Lake Shore"() -> (w985:refnum<visa-resource-name>)
                              n499 = VISA Write(VISA resource name=w985, write buffer="RANGE,1,0", error in (no error)=w984) -> (error out=w983:errorcluster)  [unwired: 2 out]
                            }
                            frame #1 {
                              n500 = call "ips_switchHeaterOff.vi"("Instrument address"=w988, "Rate"=2.0) -> ()  [unwired: 1 out]
                            }
                            frame #2 {
                              n501 = call "GPIB - BusCommand.vi"("Command"="H0", "Address"=w989) -> ()  [unwired: 2 out]
                            }
                          }
                          n502 = local write "Record ALL"(FALSE ("Record ALL")) -> ()
                          "Finished" <- TRUE
                        }
                        frame True {
                          n503 = local write "i"(w992) -> ()
                        }
                      }
                    }
                    frame True {
                      n504 = local write "j"(w994) -> ()
                    }
                  }
                }
                frame #3 {
                  # "Set rates"
                  n505 = local read "Temp/Magnetic Field"() -> (w998:bool)
                  n506 = local read "Max count array"() -> (w997:i32[])
                  n507 = local read "j"() -> (w1000:i32)
                  n508 = case shown="True" w998 {
                    tunnel: w1001 -> [w1006 _]
                    tunnel: w996 -> [w1002 w1013]
                    tunnel: [w1002 w1012] -> w995
                    frame False {
                      n509 = local read "Sweep Rate Array"() -> (w1005:dbl[])
                      n510 = local read "j"() -> (w1004:i32)
                      n511 = Index Array(array=w1005, index=w1004) -> (element=w1003:dbl)
                      n512 = Number To Fractional String(number=w1003, precision (6)=i16 3) -> (F-format string=w1009:string)  [unwired: 2 in]
                      n513 = Concatenate Strings("T" ("format string"), w1009) -> (w1010:string)
                      n514 = call "GPIB - BusCommand.vi"("Command"=w1010, "Address"=w1006) -> ()  [unwired: 2 out]
                      n515 = local write "Sweep Rate (T/min)"(w1003) -> ()
                    }
                    frame True {
                      n516 = local read "T Sweep Rate Array"() -> (w1019:dbl[])
                      n517 = local read "j"() -> (w1020:i32)
                      n518 = Index Array(array=w1019, index=w1020) -> (element=w1015:dbl)
                      n519 = Number To Fractional String(number=w1015, precision (6)=i16 1) -> (F-format string=w1017:string)  [unwired: 2 in]
                      n520 = local read "Lake Shore"() -> (w1011:refnum<visa-resource-name>)
                      n521 = local write "Temp Ramping Rate (K/min)"(w1015) -> ()
                      n522 = Concatenate Strings("RAMP 1,1," ("string"), w1017) -> (w1018:string)
                      n523 = VISA Write(VISA resource name=w1011, write buffer=w1018, error in (no error)=w1013) -> (error out=w1012:errorcluster)  [unwired: 2 out]
                    }
                  }
                  n524 = Index Array(array=w997, index=w1000) -> (element=w999:i32)
                  n525 = local write "Max Countl"(w999) -> ()
                }
                frame #4 {
                  # "Set temperature/Field"
                  n526 = local read "Temp/Magnetic Field"() -> (w1022:bool)
                  n527 = case shown="True" w1022 {
                    tunnel: [w1024 w1031] -> w1023
                    tunnel: w1021 -> [w1025 w1030]
                    frame True {
                      n528 = local read "Magnetic Field array (T)"() -> (w1028:dbl[])
                      n529 = local read "i"() -> (w1029:i32)
                      n530 = Index Array(array=w1028, index=w1029) -> (element=w1026:dbl)
                      n531 = call "Set_B.vi"("error in (no error)"=w1025, "address string"="25", "Set Field (T)"=w1026) -> ("error out"=w1024:errorcluster)  [unwired: 8 in]
                    }
                    frame False {
                      n532 = local read "Temperature Array"() -> (w1034:dbl[])
                      n533 = local read "i"() -> (w1033:i32)
                      n534 = Index Array(array=w1034, index=w1033) -> (element=w1032:dbl)
                      n535 = local read "Lake Shore"() -> (w1036:refnum<visa-resource-name>)
                      n536 = Number To Fractional String(number=w1032, precision (6)=i16 3) -> (F-format string=w1037:string)  [unwired: 2 in]
                      n537 = Concatenate Strings("SETP 1," ("write buffer"), w1037) -> (w1039:string)
                      n538 = VISA Write(VISA resource name=w1036, write buffer=w1039, error in (no error)=w1030) -> (error out=w1031:errorcluster)  [unwired: 2 out]
                    }
                  }
                }
                frame #5 {
                  n539 = local read "Finished"() -> (w1042:bool)
                  n540 = case shown="False" w1042 {
                    tunnel: [w1071 w1104] -> w1043
                    tunnel: w1041 -> [_ _]
                    tunnel: w1040 -> [w1068 w1104]
                    frame False {
                      w1066 = "_" ("string")
                      # "Wait, create Files"
                      n541 = local read "Magnetic Field array (T)"() -> (w1053:dbl[])
                      n542 = local read "Temp/Magnetic Field"() -> (w1045:bool)
                      n543 = local read "Temperature Array"() -> (w1058:dbl[])
                      n544 = local read "T Sweep Rate Array"() -> (w1055:dbl[])
                      n545 = local read "Sweep Rate Array"() -> (w1056:dbl[])
                      n546 = local read "i"() -> (w1094:i32)
                      n547 = local read "j"() -> (w1092:i32)
                      n548 = Select(t=w1055, s=w1045, f=w1056) -> (s? t:f=w1054:dbl[])
                      n549 = Index Array(array=w1054, index=w1092) -> (element=w1063:dbl)
                      n550 = Round Toward -Infinity(1:w1063) -> (0:w1064:dbl)
                      n551 = Multiply(x=w1053, y=i16 1000 ("precision (6)")) -> (x*y=w1051:dbl[])
                      n552 = Select(t=w1051, s=w1045, f=w1058) -> (s? t:f=w1057:dbl[])
                      n553 = Index Array(array=w1057, index=w1094) -> (element=w1093:dbl)
                      n554 = Number To Fractional String(use system decimal point (T)=TRUE, number=w1093, precision (6)=i16 1) -> (F-format string=w1095:string)  [unwired: 1 in]
                      n555 = Subtract(x=w1063, y=w1064) -> (x-y=w1065:dbl)
                      n556 = Equal To 0?(x=w1065) -> (x = 0?=w1062:bool)
                      n557 = Select(t="mT" ("string"), s=w1045, f="K" ("string")) -> (s? t:f=w1048:string)
                      n558 = Select(t=i16 0 ("precision (6)"), s=w1062, f=i16 2 ("precision (6)")) -> (s? t:f=w1059:i16)
                      n559 = Number To Fractional String(use system decimal point (T)=TRUE, number=w1063, precision (6)=w1059) -> (F-format string=w1067:string)  [unwired: 1 in]
                      n560 = Select(t="Kpm" ("string"), s=w1045, f="Tpm" ("string")) -> (s? t:f=w1044:string)
                      n561 = Concatenate Strings("Directory", "\\" ("string"), "FileName", w1066, w1095, w1048, w1066, w1067, w1044) -> (w1088:string)
                      n562 = Search and Replace String(replace all?=TRUE ("replace all? (F)"), input string=w1088, search string=".", replace string="p" ("substring (\"\")"), error in=w1068) -> (result string=w1083:string, error out=w1078:errorcluster)  [unwired: 3 in, 2 out]
                      n563 = local write "Step Rate"(FALSE ("Step Rate")) -> ()
                      n564 = Concatenate Strings(w1083, ".txt" ("string")) -> (w1082:string)
                      n565 = local read "Step Temp"() -> (w1072:bool)
                      n566 = String To Path(string=w1082) -> (path=w1081:path)
                      n567 = Open/Create/Replace File(file path (use dialog)=w1081, error in=w1078, operation (0:open)=T5."open or create") -> (refnum out=w1070:refnum<file>, error out=w1071:errorcluster)  [unwired: 3 in, 1 out]
                      n568 = local write "refnum out"(w1070) -> ()
                      n569 = Refnum to Path(1:w1070) -> (0:w1073:path)
                      n570 = call "Create_sweep_files.vi"("Measurement File"=w1073) -> ("Path 3"=w1076:path, "Path 2"=w1075:path, "Path"=w1074:path)  [unwired: 8 in]
                      n571 = local write "Measurement File"(w1073) -> ()
                      n572 = case shown="True" w1072 {
                        frame False {
                        }
                        frame True {
                          n573 = Get Date/Time In Seconds() -> (seconds since 1Jan1904=w1097:timestamp)
                          n574 = local write "Step Temp"(FALSE ("Step Temp")) -> ()
                          n575 = while {
                            tunnel: w1097 -> [w1102]
                            stop <- w1099 stop-if-true
                            n576 = Get Date/Time In Seconds() -> (seconds since 1Jan1904=w1103:timestamp)
                            n577 = Subtract(x=w1103, y=w1102) -> (x-y=w1101:dbl)
                            "Wait (s)" <- w1101
                            n578 = Greater Or Equal?(x=w1101, y="secs to wait") -> (x >= y?=w1099:bool)
                          }
                        }
                      }
                      n579 = local write "Measurement File_dn"(w1076) -> ()
                      n580 = local write "Measurement File_average"(w1074) -> ()
                      n581 = local write "Measurement File_up"(w1075) -> ()
                    }
                    frame True {
                    }
                  }
                }
                frame #6 {
                  n582 = local read "Finished"() -> (w1105:bool)
                  n583 = case shown="True" w1105 {
                    frame False {
                      n584 = local write "Measuring"(TRUE ("Measuring")) -> ()
                    }
                    frame True {
                      n585 = local write "Measure /Pause"(FALSE ("Measure /Pause")) -> ()
                    }
                  }
                }
              }
            }
            frame "Return" {
            }
          }
        }
      }
      frame Error {
        # "Return true for any case which should stop the loop."
      }
    }
  }
  n586 = VISA Read(VISA resource name=w21, byte count=u32 100, error in (no error)=w23) -> (VISA resource name out=w20:refnum<visa-resource-name>, read buffer=w19:string, error out=w22:errorcluster)  [unwired: 1 out]
  n587 = VISA Open(error in (no error)=w22, VISA resource name="Magnetic Field") -> (VISA resource name=w115:refnum<visa-resource-name>, error out=w97:errorcluster)  [unwired: 3 in]
  n588 = VISA Open(error in (no error)=w97, VISA resource name="Lake Shore") -> (VISA resource name=w92:refnum<visa-resource-name>, error out=w62:errorcluster)  [unwired: 3 in]
  n589 = VISA Write(VISA resource name="Lake Shore", write buffer="KRDG?a", error in (no error)=w62) -> (VISA resource name out=w59:refnum<visa-resource-name>, error out=w58:errorcluster)  [unwired: 1 out]
  n590 = VISA Read(VISA resource name=w59, byte count=w65, error in (no error)=w58) -> (VISA resource name out=w56:refnum<visa-resource-name>, read buffer=w70:string, error out=w57:errorcluster)  [unwired: 1 out]
  n591 = VISA Write(VISA resource name=w56, write buffer="SETP?a", error in (no error)=w57) -> (VISA resource name out=w55:refnum<visa-resource-name>, error out=w54:errorcluster)  [unwired: 1 out]
  n592 = VISA Read(VISA resource name=w55, byte count=w65, error in (no error)=w54) -> (VISA resource name out=w52:refnum<visa-resource-name>, read buffer=w69:string, error out=w53:errorcluster)  [unwired: 1 out]
  n593 = VISA Write(VISA resource name=w52, write buffer="RANGE?a", error in (no error)=w53) -> (VISA resource name out=w50:refnum<visa-resource-name>, error out=w51:errorcluster)  [unwired: 1 out]
  n594 = Fract/Exp String To Number(string=w70) -> (number=w68:dbl)  [unwired: 3 in, 1 out]
  n595 = VISA Read(VISA resource name=w50, byte count=w65, error in (no error)=w51) -> (read buffer=w64:string, error out=w61:errorcluster)  [unwired: 2 out]
  n596 = Fract/Exp String To Number(string=w69) -> (number=w67:dbl)  [unwired: 3 in, 1 out]
  n597 = Fract/Exp String To Number(string=w64) -> (number=w60:dbl)  [unwired: 3 in, 1 out]
  n598 = local write "Actual Temperature (K)"(w68) -> ()
  n599 = local write "Setpoint Temperature (K)"(w67) -> ()
  n600 = local write "Heater Range"(w60) -> ()
  n601 = case shown="True" w75 {
    frame False {
    }
    frame True {
      n602 = invoke on="P(T)" class="XYGraph (strict)" method="Reinit To Default"() -> ()  [unwired: 3 in, 3 out]
      n603 = invoke on="I(T)" class="XYGraph (strict)" method="Reinit To Default"() -> ()  [unwired: 3 in, 3 out]
    }
  }
  n604 = Decimal String To Number(string=w19) -> (number=w18:i32)  [unwired: 2 in, 1 out]
  n605 = local write "Keithley (IV conv) averaging"(w18) -> ()
  n606 = while {
    shift-right: [w1136] -> w113
    shift-left: w94 -> [w1137]
    shift-right: [w1138] -> w118
    shift-left: w119 -> [w1139]
    tunnel: w20 -> [w1135]
    tunnel: w115 -> [w1134]
    tunnel: w61 -> [_]
    tunnel: [w1128] -> _
    tunnel: w102 -> [w1127]
    tunnel: w92 -> [w1126]
    tunnel: w28 -> [w1125]
    stop <- "stop" stop-if-true
    n607 = event shown="[0] Timeout" {
      selector: _ -> [_ _ _ _ _ _ _ _ _ _ _ _ _ _ _ _]
      dyn-events: _ -> [_ _ _ _ _ _ _ _ _ _ _ _ _ _ _ _]
      timeout: 10 -> [_ _ _ _ _ _ _ _ _ _ _ _ _ _ _ _]
      tunnel: w1139 -> [w1149 w1195 w1213 w1223 w1237 w1308 w1312 w1316 w1372 w1388 w1405 w1448 w1465 w1489 w1491 w1502]
      tunnel: [w1148 w1195 w1213 w1223 w1237 w1308 w1312 w1316 w1372 w1388 w1405 w1448 w1465 w1489 w1491 w1502] -> w1138
      tunnel: w1137 -> [w1147 w1204 w1212 w1222 w1235 w1307 w1314 w1318 w1373 w1387 w1404 w1449 w1467 w1483 w1495 w1504]
      tunnel: [w1146 w1196 w1212 w1222 w1234 w1309 w1314 w1317 _ w1387 w1404 w1449 w1466 w1482 w1494 w1503] -> w1136
      tunnel: w1135 -> [w1145 w1205 _ _ _ _ _ _ _ _ _ _ _ _ _ _]
      tunnel: w1134 -> [w1144 _ _ _ _ _ _ _ _ _ _ _ _ _ _ _]
      tunnel: [w1142 w1194 w1211 w1221 w1236 w1310 w1313 w1315 w1371 w1386 w1403 w1447 w1464 w1490 w1492 _] -> w1128
      tunnel: w1127 -> [w1142 w1194 w1211 w1224 w1236 w1310 w1313 w1315 w1371 w1386 w1403 w1447 w1464 w1490 w1492 _]
      tunnel: w1126 -> [_ _ _ _ _ _ _ _ _ _ _ _ w1468 w1481 w1496 w1501]
      tunnel: [_ _ _ _ _ _ _ _ w1373 _ _ _ _ _ _ _] -> _
      tunnel: w1125 -> [w1141 _ _ _ _ _ _ _ _ _ _ _ _ _ _ _]
      event Timeout {
        n608 = event-data() -> ()  [unwired: 1 in, 3 out]
        n609 = case shown="True" "Measuring" {
          tunnel: w1149 -> [w1151 w1174]
          tunnel: [w1151 w1173] -> w1148
          tunnel: w1147 -> [w1150 w1152]
          tunnel: [w1150 w1172] -> w1146
          tunnel: w1145 -> [_ w1165]
          tunnel: w1144 -> [_ w1164]
          tunnel: w1141 -> [_ w1155]
          frame False {
          }
          frame True {
            w1163 = ":FETCh? " ("data")
            w1166 = u32 1000 ("byte count")
            # "Generate the data here."
            n610 = case shown="No Error" w1152 {
              selector: w1152 -> [w1186 w1187]
              tunnel: [w1186 w1187] -> w1160
              tunnel: [w1185 _] -> w1159
              frame No Error {
                n611 = Get Date/Time In Seconds() -> (seconds since 1Jan1904=w1185:timestamp)
              }
              frame Error {
              }
            }
            n612 = VISA Write(VISA resource name=w1165, write buffer=w1163, error in (no error)=w1160) -> (VISA resource name out=w1171:refnum<visa-resource-name>, error out=w1169:errorcluster)  [unwired: 1 out]
            n613 = VISA Write(VISA resource name=w1164, write buffer=w1163, error in (no error)=w1169) -> (VISA resource name out=w1170:refnum<visa-resource-name>, error out=w1168:errorcluster)  [unwired: 1 out]
            n614 = VISA Read(VISA resource name=w1171, byte count=w1166, error in (no error)=w1168) -> (read buffer=w1161:string, error out=w1167:errorcluster)  [unwired: 2 out]
            n615 = VISA Read(VISA resource name=w1170, byte count=w1166, error in (no error)=w1167) -> (read buffer=w1162:string, error out=w1157:errorcluster)  [unwired: 2 out]
            n616 = case shown="False" "DaQ" {
              tunnel: w1157 -> [w1176 w1182]
              tunnel: [w1176 w1181] -> w1156
              tunnel: w1155 -> [_ w1180]
              tunnel: [0.0 ("Output") w1178] -> w1153
              frame False {
              }
              frame True {
                n617 = local read "Number of Samples"() -> (w1184:i32)
                n618 = call-poly <vilib>:"DAQmx Read.vi"("task/channels in"=w1180, "number of samples per channel"=w1184, "error in"=w1182) -> ("data"=w1183:dbl[], "error out"=w1181:errorcluster)  [unwired: 10 in, 1 out]
                n619 = call-poly <vilib>:"Mean.vi"("X"=w1183) -> ("mean"=w1179:dbl)  [unwired: 1 out]
                "Actual mean" <- w1179
                n620 = call "N Point Running Average.vi"("n"="Moving average", "Input"=w1179) -> ("Output"=w1178:dbl)
              }
            }
            n621 = Bundle("seconds since 1Jan1904"=w1159, "read buffer"=w1161, "read buffer"=w1162, "Output"=w1153) -> (w1158:T4)  [unwired: 1 in]
            n622 = Enqueue Element(queue=w1174, element=w1158, error in (no error)=w1156) -> (queue out=w1173:refnum<queue>, error out=w1172:errorcluster)  [unwired: 1 in, 1 out]
          }
        }
      }
      event "Keithley (IV conv) averaging": Value Change {
        n623 = event-data() -> ()  [unwired: 1 in, 6 out]
        n624 = Number To Decimal String(number="Keithley (IV conv) averaging") -> (decimal integer string=w1202:string)  [unwired: 1 in]
        n625 = Concatenate Strings("VOLTage:DC:AVERage:COUNt " ("write buffer"), w1202) -> (w1201:string)
        n626 = VISA Write(VISA resource name=w1205, write buffer=w1201, error in (no error)=w1204) -> (VISA resource name out=w1200:refnum<visa-resource-name>, error out=w1198:errorcluster)  [unwired: 1 out]
        n627 = VISA Write(VISA resource name=w1200, write buffer="VOLTage:DC:AVERage:COUNt?", error in (no error)=w1198) -> (VISA resource name out=w1193:refnum<visa-resource-name>, error out=w1197:errorcluster)  [unwired: 1 out]
        n628 = VISA Read(VISA resource name=w1193, byte count=u32 100, error in (no error)=w1197) -> (read buffer=w1191:string, error out=w1196:errorcluster)  [unwired: 2 out]
        n629 = Decimal String To Number(string=w1191) -> (number=w1190:i32)  [unwired: 2 in, 1 out]
        n630 = Equal?(x="Keithley (IV conv) averaging", y=w1190) -> (x = y?=→"Confirm":bool)
      }
      event "Max Field (T)": Value Change {
        n631 = event-data() -> ()  [unwired: 1 in, 6 out]
        n632 = Divide(x="Max Field (T)", y="dB (T)") -> (x/y=w1208:dbl)
        n633 = for {
          N: w1208 -> [_]
          tunnel: "dB (T)" -> [w1218]
          tunnel: [w1215] -> w1207 mode=indexing
          tunnel: "Min Field (T)" -> [w1216]
          tunnel: [0.0] -> _ mode=indexing
          i -> [w1219]
          n634 = Multiply(x=w1219, y=w1218) -> (x*y=w1217:dbl)
          n635 = Add(x=w1217, y=w1216) -> (x+y=w1215:dbl)
        }
        "B array" <- w1207
      }
      event "Sweep Rate (T/min)": Value Change {
        n636 = event-data() -> ("NewVal"=w1225:dbl)  [unwired: 1 in, 5 out]
        n637 = local read "Magnet"() -> (w1220:bool)
        n638 = case shown="False" w1220 {
          tunnel: w1225 -> [_ w1232]
          tunnel: w1224 -> [w1226 w1228]
          tunnel: [w1226 w1227] -> w1221
          frame False {
          }
          frame True {
            n639 = Number To Fractional String(number=w1232, precision (6)=i16 3) -> (F-format string=w1230:string)  [unwired: 2 in]
            n640 = Concatenate Strings("T" ("format string"), w1230) -> (w1229:string)
            n641 = call "GPIB - BusCommand.vi"("Command"=w1229, "Address"=w1228) -> ("Address(thru)"=w1227:T6)  [unwired: 1 out]
          }
        }
      }
      event "Field To Zero": Value Change {
        n642 = event-data() -> ()  [unwired: 1 in, 6 out]
        n643 = Two Button Dialog(message="Do you want to switch off the field?", 1:"No" ("F button name (\"Cancel\")"), 2:"Yes" ("T button name (\"OK\")")) -> (T button?=w1241:bool)
        n644 = case shown="True" w1241 {
          tunnel: w1236 -> [_ w1246]
          tunnel: w1235 -> [w1242 w1244]
          tunnel: [w1242 w1243] -> w1234
          frame False {
          }
          frame True {
            n645 = local read "Magnet"() -> (w1245:bool)
            n646 = case shown="False" w1245 {
              tunnel: w1246 -> [_ w1298]
              tunnel: w1244 -> [w1249 w1295]
              tunnel: [w1248 w1295] -> w1243
              frame False {
                n647 = local read "Lock_in_Amplifier"() -> (w1247:refnum<visa-resource-name>)
                n648 = stacked-sequence {
                  seq-local: [w1252 _] -> [_ w1264]
                  seq-local: [w1250 _] -> [_ w1261]
                  tunnel: w1249 -> [w1254 _]
                  tunnel: [_ w1267] -> w1248
                  tunnel: w1247 -> [w1251 w1262]
                  frame #0 {
                    n649 = VISA Write(VISA resource name=w1251, write buffer="AUXV?1", error in (no error)=w1254) -> (VISA resource name out=w1258:refnum<visa-resource-name>, error out=w1253:errorcluster)  [unwired: 1 out]
                    n650 = VISA Read(VISA resource name=w1258, byte count=u32 1000, error in (no error)=w1253) -> (read buffer=w1255:string, error out=w1252:errorcluster)  [unwired: 2 out]
                    n651 = Fract/Exp String To Number(string=w1255) -> (number=w1250:dbl)  [unwired: 3 in, 1 out]
                  }
                  frame #1 {
                    w1270 = 0.001 ("Voltage Step (V)")
                    n652 = local read "Sweep Rate (T/min)"() -> (w1269:dbl)
                    n653 = local read "V/I (Ohm)"() -> (w1266:dbl)
                    n654 = local read "B/V (T/V)"() -> (w1260:dbl)
                    n655 = xnode "Sweep Delay"("SweepRate"=w1269, "Resolution"=w1270, "BpV"=w1260) -> ("Result"=w1268:dbl)  [unwired: 1 in, 1 out]
                    n656 = call "Universal_Ramping.vi"("milliseconds to wait"=w1268, "Initial Voltage (V)"=w1261, "error in (no error)"=w1264, "Voltage Step (V)"=w1270, "Final Voltage (V)"=0.0, "VISA resource name"=w1262) -> ("error out"=w1267:errorcluster, "Actual Voltage (V)"=w1259:dbl)  [unwired: 3 in, 1 out]
                    n657 = local write "Actual Voltage (V)"(w1259) -> ()
                    n658 = xnode "AUXtoB"("BpV"=w1260, "Rm"=w1266, "Aux"=w1259) -> ("Result"=w1265:dbl)  [unwired: 1 in, 1 out]
                    n659 = local write "Actual B Field (T)"(w1265) -> ()
                  }
                }
              }
              frame True {
                n660 = local read "Sweep Rate (T/min)"() -> (w1297:dbl)
                n661 = call "ips_switchHeaterOff.vi"("Instrument address"=w1298, "Rate"=w1297) -> ("B"=w1296:dbl)
                n662 = local write "Actual Field (T)"(w1296) -> ()
              }
            }
          }
        }
      }
      event "Go to Set": Value Change {
        n663 = event-data() -> ()  [unwired: 1 in, 6 out]
        n664 = local read "V/I (Ohm)"() -> (w1305:dbl)
        n665 = local read "B/V (T/V)"() -> (w1304:dbl)
        n666 = local read "Lock_in_Amplifier"() -> (w1301:refnum<visa-resource-name>)
        n667 = local read "Sweep Rate (T/min)"() -> (w1303:dbl)
        n668 = local read "Magnet"() -> (w1306:bool)
        n669 = call "Ramp_Field.vi"("Set Field (T) in"="Set Field (T)", "Sweep Rate (T/min)"=w1303, "V/I (Ohm)"=w1305, "error in (no error)"=w1307, "Magnet"=w1306, "B/V (T/V)"=w1304, "VISA Refnum in"=w1301) -> ("error out"=w1309:errorcluster, "Actual Voltage (V)"=w1299:dbl, "Set Field (T) out"=w1302:dbl)  [unwired: 2 in]
        n670 = local write "Actual B Field (T)"(w1302) -> ()
        n671 = local write "Actual Voltage (V)"(w1299) -> ()
      }
      event "Measure /Pause": Value Change {
        n672 = event-data() -> ("NewVal"=w1311:bool)  [unwired: 1 in, 5 out]
        n673 = local write "Measuring"(w1311) -> ()
      }
      event "Stop": Value Change {
        n674 = event-data() -> ()  [unwired: 1 in, 6 out]
        n675 = local read "Measuring"() -> (w1319:bool)
        n676 = case shown="True" w1319 {
          tunnel: w1318 -> [w1320 w1322]
          tunnel: [w1320 w1323] -> w1317
          frame False {
          }
          frame True {
            w1324 = FALSE ("Measuring")
            n677 = local read "Temp/Magnetic Field"() -> (w1321:bool)
            n678 = local read "SaveSweep"() -> (w1325:bool)
            n679 = local write "Measuring"(w1324) -> ()
            n680 = local write "Measure /Pause"(w1324) -> ()
            n681 = case shown="False" w1321 {
              tunnel: [w1329 w1338] -> w1323
              tunnel: w1322 -> [w1328 w1339]
              frame False {
                n682 = local read "Lock_in_Amplifier"() -> (w1330:refnum<visa-resource-name>)
                n683 = local read "V/I (Ohm)"() -> (w1334:dbl)
                n684 = local read "Sweep Rate (T/min)"() -> (w1333:dbl)
                n685 = local read "Set Field (T)"() -> (w1335:dbl)
                n686 = local read "B/V (T/V)"() -> (w1331:dbl)
                n687 = local read "Magnet"() -> (w1332:bool)
                n688 = call "Ramp_Field.vi"("Set Field (T) in"=w1335, "Sweep Rate (T/min)"=w1333, "V/I (Ohm)"=w1334, "error in (no error)"=w1328, "Magnet"=w1332, "B/V (T/V)"=w1331, "VISA Refnum in"=w1330) -> ("error out"=w1329:errorcluster, "Actual Voltage (V)"=w1326:dbl, "Set Field (T) out"=w1327:dbl)  [unwired: 2 in]
                n689 = local write "Actual B Field (T)"(w1327) -> ()
                n690 = local write "Actual Voltage (V)"(w1326) -> ()
              }
              frame True {
                n691 = local read "Set temperature (K)"() -> (w1336:dbl)
                n692 = Number To Fractional String(number=w1336, precision (6)=i16 3) -> (F-format string=w1342:string)  [unwired: 2 in]
                n693 = local read "Lake Shore"() -> (w1337:refnum<visa-resource-name>)
                n694 = Concatenate Strings("SETP 1," ("write buffer"), w1342) -> (w1340:string)
                n695 = VISA Write(VISA resource name=w1337, write buffer=w1340, error in (no error)=w1339) -> (error out=w1338:errorcluster)  [unwired: 2 out]
              }
            }
            n696 = case shown="True" w1325 {
              tunnel: w1321 -> [_ w1344]
              frame False {
              }
              frame True {
                w1351 = 1 ("index (row)")
                w1352 = 0 ("index (row)")
                n697 = case shown="True" w1344 {
                  tunnel: [w1368 w1370] -> w1362
                  tunnel: [w1367 w1369] -> w1345
                  frame True {
                    n698 = local read "Averaged P(T)"() -> (w1367:dbl[][])
                    n699 = local read "I(T) /Averaged/"() -> (w1368:cluster{"B array":dbl[], dbl[]}[])
                  }
                  frame False {
                    n700 = local read "Averaged P(B)"() -> (w1369:dbl[][])
                    n701 = local read "I(B) /Averaged/"() -> (w1370:cluster{"B array":dbl[], dbl[]}[])
                  }
                }
                n702 = local read "Measurement File_average"() -> (w1363:path)
                n703 = local read "Averaged dt"() -> (w1354:dbl[][])
                n704 = Index Array(array=w1354, index (row)=w1352) -> (element=w1353:dbl[])  [unwired: 1 in]
                n705 = Index Array(array=w1354, index (row)=w1351) -> (element=w1347:dbl[])  [unwired: 1 in]
                n706 = Index Array(array=w1362, index=1) -> (element=w1358:cluster{"B array":dbl[], dbl[]})
                n707 = Index Array(array=w1362, index=0) -> (element=w1359:cluster{"B array":dbl[], dbl[]})
                n708 = Unbundle(w1358) -> ("B array"=w1349:dbl[], w1348:dbl[])
                n709 = Unbundle(w1359) -> ("B array"=w1357:dbl[], w1356:dbl[])
                n710 = Index Array(array=w1345, index (row)=w1352) -> (element=w1350:dbl[])  [unwired: 1 in]
                n711 = Index Array(array=w1345, index (row)=w1351) -> (element=w1346:dbl[])  [unwired: 1 in]
                n712 = Build Array(w1357, w1356, w1353, w1350, w1349, w1348, w1347, w1346) -> (w1355:dbl[][])
                n713 = call-poly <vilib>:"Write Delimited Spreadsheet.vi"("file path (dialog if empty)"=w1363, "format (%.3f)"="%.5g", "2D data"=w1355, "append to file? (F)"=TRUE ("transpose? (F)"), "transpose? (F)"=TRUE ("append to file? (F)")) -> ()  [unwired: 9 in, 2 out]
              }
            }
          }
        }
      }
      event "Sweep": Value Change {
        n714 = event-data() -> ("NewVal"=w1374:bool)  [unwired: 1 in, 5 out]
        n715 = case shown="True" w1374 {
          frame False {
          }
          frame True {
            n716 = local read "Measurement File"() -> (w1375:path)
            n717 = Two Button Dialog(message="Do you want to create additional files for the sweeping measurements?" ("string"), 1:"No" ("F button name (\"Cancel\")"), 2:"Yes" ("T button name (\"OK\")")) -> (T button?=w1377:bool)
            n718 = case shown="True" w1377 {
              tunnel: w1375 -> [_ w1382]
              frame False {
                n719 = local write "SaveSweep"(FALSE ("SaveSweep")) -> ()
              }
              frame True {
                n720 = call "Create_sweep_files.vi"("Measurement File"=w1382) -> ("Path 3"=→"Measurement File_dn":path, "Path 2"=→"Measurement File_up":path, "Path"=→"Measurement File_average":path)  [unwired: 8 in]
                "SaveSweep" <- TRUE
              }
            }
          }
        }
      }
      event "Measure Noise": Value Change {
        n721 = event-data() -> ("NewVal"=w1389:bool)  [unwired: 1 in, 5 out]
        n722 = case shown="True" w1389 {
          frame False {
          }
          frame True {
            n723 = local read "Gain (V/A)"() -> (w1394:dbl)
            n724 = call "Noise_measurement.vi"("Gain (V/A)"=w1394, "Cycles"="Cycles", "Lower Cut-Off"="Cut-Off Frequency", "minimum value"="minimum value", "Filter On"="Filter On", "maximum value"="maximum value", "physical channels"="physical channels", "rate"="Rate", "samples per channel"="Samples per channel") -> ("Current (pA) Filtered"=→"Current (pA) Filtered":waveform(dbl), "PSD (pA/Hz^1/2) Peaks Removed"=→"PSD (pA/Hz^1/2) Peaks Removed":cluster{"f0":dbl, "df":dbl, "magnitude":dbl[]}, "Current (pA)"=→"Current (pA)":dbl[], "PSD (pA/Hz^1/2)"=→"PSD (pA/Hz^1/2)":cluster{"f0":dbl, "df":dbl, "magnitude":dbl[]})  [unwired: 3 in]
          }
        }
      }
      event "Calibrate": Value Change {
        n725 = event-data() -> ()  [unwired: 1 in, 6 out]
        n726 = case shown="True" "Calibrate" {
          frame False {
          }
          frame True {
            w1409 = dbl[] []
            n727 = while {
              shift-right: [w1442] -> w1407
              shift-left: dbl[][] [] -> [w1441]
              shift-right: [w1425] -> _
              shift-left: w1409 -> [w1437]
              shift-right: [w1434] -> _
              shift-left: w1409 -> [w1436]
              shift-right: [w1424] -> _
              shift-left: w1409 -> [w1435]
              shift-right: [w1416] -> _
              shift-left: 0.0 ("Set Field out") -> [w1415]
              stop <- w1438 stop-if-true
              n728 = call "Calibtarion.vi"("Dwell Time (ms)"="Dwell Time (ms)", "V array in (V)"=w1437, "I array in (A)"=w1435, "Collected array in"=w1441, "B array in (T)"=w1436, "Set Field (T)"=w1415, "dB"="dB") -> ("Best Linear Fit"=w1426:dbl[], "appended array"=→"appended array":dbl[][], "slope"=→"B/V (T/V)":dbl, "V array out (V)"=w1425:dbl[], "Boolean"=w1440:bool, "I array out (A)"=w1424:dbl[], "intercept 2"=→"I0 (A)":dbl, "Collected array out"=w1442:dbl[][], "intercept"=→"B0 (T)":dbl, "B array Out"=w1434:dbl[], "slope 2"=→"V/I (Ohm)":dbl, "Best Linear Fit 2"=w1431:dbl[], "Set Field out"=w1416:dbl)
              n729 = Bundle("I array out (A)"=w1424, "V array out (V)"=w1425) -> (w1433:T15)  [unwired: 1 in]
              n730 = Bundle("I array out (A)"=w1424, "Best Linear Fit"=w1426) -> (w1427:T16)  [unwired: 1 in]
              n731 = Bundle("V array out (V)"=w1425, "B array Out"=w1434) -> (w1429:T17)  [unwired: 1 in]
              n732 = Bundle("V array out (V)"=w1425, "Best Linear Fit 2"=w1431) -> (w1430:T18)  [unwired: 1 in]
              n733 = Or(x=w1440, y="stop 2") -> (x .or. y?=w1438:bool)
              n734 = Build Array(w1433, w1427) -> (→"V_I":T19)
              n735 = Build Array(w1429, w1430) -> (→"B_V":T20)
            }
            n736 = flat-sequence {
              tunnel: w1407 -> [w1413]
              frame #0 {
                n737 = Two Button Dialog(message="Do you want to save calibration file?") -> (T button?=w1412:bool)  [unwired: 2 in]
                n738 = case shown="True" w1412 {
                  tunnel: w1413 -> [_ w1414]
                  frame False {
                  }
                  frame True {
                    n739 = call-poly <vilib>:"Write Delimited Spreadsheet.vi"("2D data"=w1414) -> ()  [unwired: 13 in, 2 out]
                  }
                }
              }
            }
          }
        }
      }
      event "New Measurement File": Value Change {
        n740 = event-data() -> ()  [unwired: 1 in, 6 out]
        n741 = local read "Sweep"() -> (w1444:bool)
        n742 = Open/Create/Replace File(prompt="Please select measurement file\n", operation (0:open)=T5."replace or create with confirmation") -> (refnum out=w1450:refnum<file>)  [unwired: 4 in, 2 out]
        n743 = local write "refnum out"(w1450) -> ()
        n744 = Refnum to Path(1:w1450) -> (0:w1445:path)
        n745 = case shown="True" w1444 {
          tunnel: w1445 -> [_ w1453]
          frame False {
          }
          frame True {
            n746 = Two Button Dialog(message="Do you want to create additional files for the sweeping measurements?" ("string"), 1:"No" ("F button name (\"Cancel\")"), 2:"Yes" ("T button name (\"OK\")")) -> (T button?=w1455:bool)
            n747 = case shown="True" w1455 {
              tunnel: w1453 -> [_ w1463]
              frame False {
                n748 = local write "SaveSweep"(FALSE ("SaveSweep")) -> ()
              }
              frame True {
                n749 = call "Create_sweep_files.vi"("Measurement File"=w1463) -> ("Path 3"=w1460:path, "Path 2"=w1461:path, "Path"=w1462:path)  [unwired: 8 in]
                n750 = local write "Measurement File_dn"(w1460) -> ()
                n751 = local write "Measurement File_average"(w1462) -> ()
                n752 = local write "Measurement File_up"(w1461) -> ()
                n753 = local write "SaveSweep"(TRUE) -> ()
              }
            }
          }
        }
        n754 = local write "Measurement File"(w1445) -> ()
        n755 = local write "Offset?"(FALSE ("Offset?")) -> ()
        n756 = local write "First?"(TRUE ("First?")) -> ()
      }
      event "Heater On/Off": Value Change {
        n757 = event-data() -> ()  [unwired: 1 in, 6 out]
        n758 = case shown="False" "Heater On/Off" {
          tunnel: w1468 -> [w1473 w1479]
          tunnel: w1467 -> [w1471 w1480]
          tunnel: [w1470 w1478] -> w1466
          frame False {
            n759 = VISA Write(VISA resource name=w1473, write buffer="RANGE,1,0", error in (no error)=w1471) -> (error out=w1470:errorcluster)  [unwired: 2 out]
          }
          frame True {
            n760 = Number To Decimal String(number="Heater Range") -> (decimal integer string=w1476:string)  [unwired: 1 in]
            n761 = Concatenate Strings("RANGE,1," ("write buffer"), w1476) -> (w1474:string)
            n762 = VISA Write(VISA resource name=w1479, write buffer=w1474, error in (no error)=w1480) -> (error out=w1478:errorcluster)  [unwired: 2 out]
          }
        }
      }
      event "Set temperature (K)": Value Change {
        n763 = event-data() -> ()  [unwired: 1 in, 6 out]
        n764 = local read "Set temperature (K)"() -> (w1484:dbl)
        n765 = Number To Fractional String(number=w1484, precision (6)=i16 3) -> (F-format string=w1487:string)  [unwired: 2 in]
        n766 = Concatenate Strings("SETP 1," ("write buffer"), w1487) -> (w1485:string)
        n767 = VISA Write(VISA resource name=w1481, write buffer=w1485, error in (no error)=w1483) -> (error out=w1482:errorcluster)  [unwired: 2 out]
      }
      event "Temp Ramping Rate (K/min)": Value Change {
        n768 = event-data() -> ()  [unwired: 1 in, 6 out]
        n769 = local read "Temp Ramping Rate (K/min)"() -> (w1493:dbl)
        n770 = Number To Fractional String(number=w1493, precision (6)=i16 1) -> (F-format string=w1499:string)  [unwired: 2 in]
        n771 = Concatenate Strings("RAMP 1,1," ("string"), w1499) -> (w1498:string)
        n772 = VISA Write(VISA resource name=w1496, write buffer=w1498, error in (no error)=w1495) -> (error out=w1494:errorcluster)  [unwired: 2 out]
      }
      event "Heater Range": Value Change {
        n773 = event-data() -> ()  [unwired: 1 in, 6 out]
        n774 = local read "Heater On/Off"() -> (w1505:bool)
        n775 = case shown="True" w1505 {
          tunnel: w1504 -> [w1506 w1511]
          tunnel: [w1506 w1510] -> w1503
          tunnel: w1501 -> [_ w1509]
          frame False {
          }
          frame True {
            n776 = local read "Heater Range"() -> (w1507:enum16{"Off", "Low", "Medium", "High"})
            n777 = Number To Decimal String(number=w1507) -> (decimal integer string=w1513:string)  [unwired: 1 in]
            n778 = Concatenate Strings("RANGE,1," ("write buffer"), w1513) -> (w1512:string)
            n779 = VISA Write(VISA resource name=w1509, write buffer=w1512, error in (no error)=w1511) -> (error out=w1510:errorcluster)  [unwired: 2 out]
          }
        }
      }
    }
    n780 = Reciprocal(x="Sampling rate (Hz)") -> (1/x=w1132:dbl)
    n781 = Multiply(x=w1132, y=1000.0) -> (x*y=w1130:dbl)
    n782 = Wait Until Next ms Multiple(millisecond multiple=w1130) -> ()  [unwired: 1 out]
  }
  n783 = local read "Max Field (T)"() -> (w83:dbl)
  n784 = local read "Min Field (T)"() -> (w85:dbl)
  n785 = local read "dB (T)"() -> (w84:dbl)
  n786 = Divide(x=w83, y=w84) -> (x/y=w86:dbl)
  n787 = for {
    N: w86 -> [_]
    tunnel: w84 -> [w1518]
    tunnel: [w1515] -> w46 mode=indexing
    tunnel: w85 -> [w1516]
    tunnel: [0.0] -> _ mode=indexing
    i -> [w1519]
    n788 = Multiply(x=w1519, y=w1518) -> (x*y=w1517:dbl)
    n789 = Add(x=w1517, y=w1516) -> (x+y=w1515:dbl)
  }
  n790 = Multiply(x=w46, y=0.0) -> (x*y=w43:dbl[])
  n791 = Array Size(array=w43) -> (size(s)=w42:i32)
  n792 = Decrement(x=w42) -> (x-1=w41:i32)
  n793 = local write "B array"(w46) -> ()
  n794 = Array Subset(array=w43, length=w41) -> (w40:dbl[])  [unwired: 1 in]
  n795 = Build Array(w43, w43) -> (w44:dbl[][])
  n796 = local read "Max temperature (K)"() -> (w13:dbl)
  n797 = local read "Min Temperature (K)"() -> (w15:dbl)
  n798 = local write "Averaged I(B)"(w44) -> ()
  n799 = Build Array(w40, w40) -> (w39:dbl[][])
  n800 = Divide(x=w13, y="dt (K)") -> (x/y=w16:dbl)
  n801 = local write "Averaged P(B)"(w39) -> ()
  n802 = local write "Averaged dt"(w39) -> ()
  n803 = for {
    N: w16 -> [_]
    tunnel: "dt (K)" -> [w1524]
    tunnel: [w1521] -> w5 mode=indexing
    tunnel: w15 -> [w1522]
    tunnel: [0.0] -> _ mode=indexing
    i -> [w1525]
    n804 = Multiply(x=w1525, y=w1524) -> (x*y=w1523:dbl)
    n805 = Add(x=w1523, y=w1522) -> (x+y=w1521:dbl)
  }
  "T array" <- w5
  n806 = Multiply(x=w5, y=0.0) -> (x*y=w4:dbl[])
  n807 = Array Size(array=w4) -> (size(s)=w8:i32)
  n808 = Decrement(x=w8) -> (x-1=w9:i32)
  n809 = Array Subset(array=w4, length=w9) -> (w10:dbl[])  [unwired: 1 in]
  n810 = Build Array(w4, w4) -> (w7:dbl[][])
  n811 = local write "Averaged I(T)"(w7) -> ()
  n812 = Build Array(w10, w10) -> (w11:dbl[][])
  n813 = local write "Averaged P(T)"(w11) -> ()
  n814 = local write "Averaged dt"(w11) -> ()
  n815 = local read "Lake Shore"() -> (w95:refnum<visa-resource-name>)
  n816 = local read "IV converter"() -> (w111:refnum<visa-resource-name>)
  n817 = local read "Magnetic Field"() -> (w110:refnum<visa-resource-name>)
  n818 = VISA Close(VISA resource name=w111, error in (no error)=w113) -> (error out=w114:errorcluster)
  n819 = VISA Close(VISA resource name=w110, error in (no error)=w114) -> (error out=w112:errorcluster)
  n820 = Release Queue(queue=w118, error in (no error)=w112) -> (error out=w108:errorcluster)  [unwired: 1 in, 2 out]
  n821 = Merge Errors(w108, w107) -> (w109:errorcluster)
  n822 = VISA Close(VISA resource name=w95, error in (no error)=w109) -> (error out=w106:errorcluster)
  n823 = local read "refnum out"() -> (w104:refnum<file>)
  n824 = Close File(refnum=w104, error in=w106) -> (error out=w105:errorcluster)  [unwired: 1 out]
  n825 = call <vilib>:"Simple Error Handler.vi"("error in (no error)"=w105) -> ()  [unwired: 4 in, 5 out]
  "i" <- w76
  "j" <- w76
